vi "SPIM Controller.v2.vi"() -> ()   [LabVIEW 2015]
uses:
  controls/Microscope Settings.ctl
  controls/CameraState.ctl
  controls/Stack_State.ctl
  controls/Stack Track.ctl
  controls/CameraControlTypeDef.ctl
  controls/ModeEnum.ctl
  controls/Hardware.ctl
  <vilib>/Waveform/DWDTOps.llb/DWDT Append Digital Samples.vi
  <vilib>/Waveform/WDTOps.llb/WDT Append Waveforms DBL.vi
  <vilib>/Waveform/WDTOps.llb/WDT Waveform Duration DBL.vi
  <vilib>/vision/NI_Vision_Development_Module.lvlib
panel:
  out "Frames":i32
  out "Number Of Cameras":u32
  out "Numeric 3":i32
  out "Numeric 2":i32
  out "Stack Number":i32
  out "Numeric":i32
  in  "Tab Control":enum32{"Camera Settings", "Recording"}(tab)
  in  "Tweezers":T1={"Start /um"=40.0, "Step/um"=5.0, "Range /um"=20.0} {"Range /um" min=0.0 max=10.0 step=0.05; "Step/um" min=0.0001 max=10.0 step=0.05; "Start /um" min=0.0 max=10.0 step=0.05}
  in  "?":bool
  in  "Advanced DCAM Controls":i32(listbox) caption="Multicolumn Listbox"
  out "Waveform Duration":string
  in  "Microscope Settings":T2={"Mode"=enum."XY", "Slit"={"Scanning Mode"=12.0, "Slit Width /%"=5.0}, "Colour"=[{"Laser"=enum."561", "Filter"=4}], "Exposure/ms"=40.0, "Piezo Position /um"=0.0, "ROI"={"X"={"Start /px"=0.0, "Step /px"=1.0, "Range /px"=2048.0}, "Y"={"Start /px"=0.0, "Step /px"=1.0, "Range /px"=2048.0}, "Z "={"Start /um"=0.0, "Step/um"=1.0, "Range /um"=100.0}, "T "={"Start /s"=0.0, "Step /s"=1.0, "Range /s"=100.0}}, "Samples per millisecond"=100.0, "Relax/ms"=10.0, "Readout Direction"=2.0, "Trigger Source"=2.0, "Camera Delay /ms"=11.0, "Under Scan /ms"=5.0, "Calibration Coordinates"={"Top Left"=[-4.418670520231216, -0.1592138728323702, 10.0], "Top Right"=[-9.501965317919073, -0.1592138728323702, 10.0], "Bottom Left"=[-4.4508670520231215, 0.0, 0.0], "Bottom Right"=[-9.53757225433526, 0.0, 0.0], "Waveforms"={"Analogue Out"=[], "Digital Out"=[]}}} {"Under Scan /ms" min=0.0 max=10.0 step=0.05; "ROI"."T"."Range /s" min=0.0 max=10.0 step=0.05 format="%<%H:%M:%S>t"; "ROI"."T"."Step /s" min=0.0 max=10.0 step=0.05 format="%<%M:%S%2u>t"; "ROI"."T"."Start /s" min=0.0 max=10.0 step=0.05 format="%<%M:%S%2u>t"; "ROI"."X"."Range /px" min=0.0 max=10.0 step=0.05; "ROI"."X"."Step /px" min=0.0 max=10.0 step=0.05; "ROI"."X"."Start /px" min=0.0 max=10.0 step=0.05; "ROI"."Y"."Range /px" min=0.0 max=10.0 step=0.05; "ROI"."Y"."Step /px" min=0.0 max=10.0 step=0.05; "ROI"."Y"."Start /px" min=0.0 max=10.0 step=0.05; "ROI"."Z"."Range /um" min=0.0 max=10.0 step=0.05; "ROI"."Z"."Step/um" min=0.0001 max=10.0 step=0.05; "ROI"."Z"."Start /um" min=0.0 max=10.0 step=0.05; "Colour"."Filter" items=["Empty"=1, ""=2, ""=3, "561"=4, ""=5, "488"=6]; "Camera Delay /ms" min=0.0 max=10.0 step=0.05; "Trigger Source" items=["Internal"=1.0, "External"=2.0]; "Readout Direction" items=["Forward"=1.0, "Backward"=2.0]; "Slit"."Scanning Mode" items=["Full Frame"=1.0, "Slit Scanning"=12.0]; "Piezo Position /um" min=0.0 max=10.0 step=0.05}
  in  "Frames":i32
  in  "Scan Continuously":bool
  in  "Scan Cont":bool
  in  "Scans":dbl=1.0 min=0.0 max=10.0 step=0.05
  in  "Scan":bool
  in  "Save to:":path=path "C:/_DATA/test.tiff"
  out "error IO":errorcluster
  in  "Multicolumn Listbox":i32(listbox)
  out "FPS":dbl
  out "Image":T3(plugin-control)
  out "Histogram":T4(graph)
  in  "stop":bool
  in  "Load Settings":bool
  in  "Save Settings":bool
  in  "Record":bool
  in  "Signals Debugger":bool
  in  "Stage Controller":bool
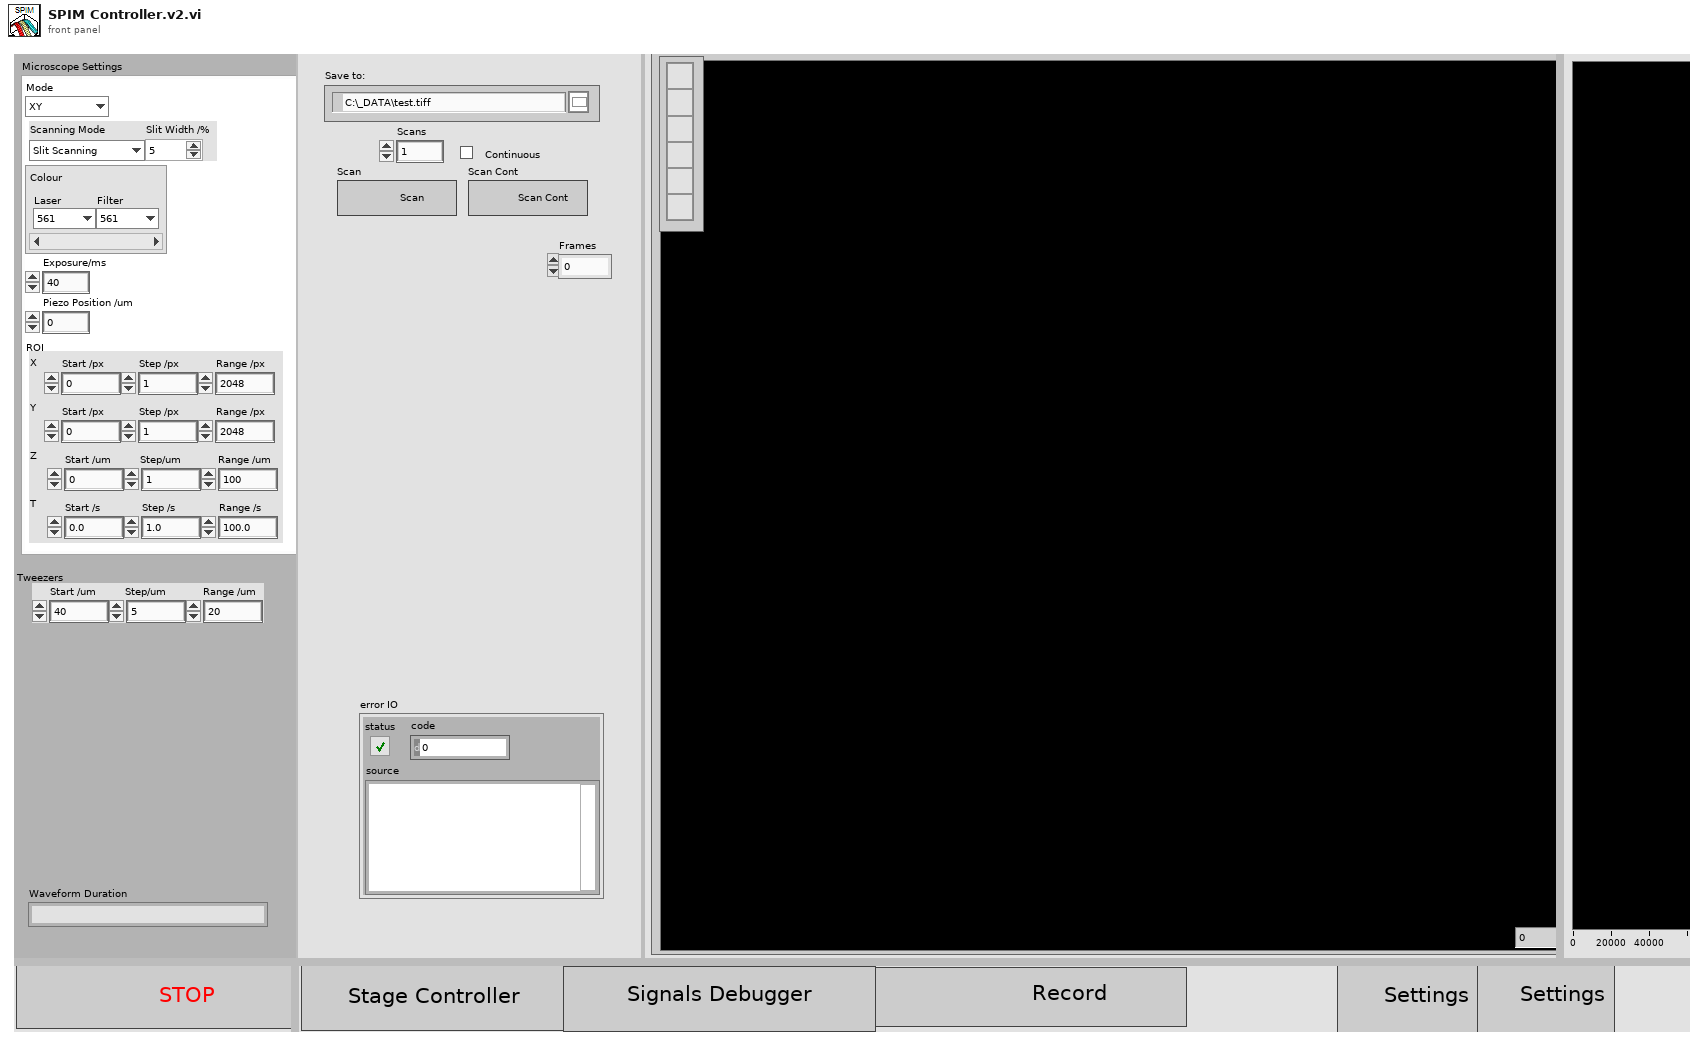
[diagram p1: front panel]
types:
  T1 = cluster{"Start /um":dbl, "Step/um":dbl, "Range /um":dbl}
  T2 = typedef "Microscope Settings.ctl" = cluster{"Mode":enum16{"X", "XY", "XYZ", "XYZT", "XYZC", "Tweezers", "Virus"}, "Slit":cluster{"Scanning Mode":dbl, "Slit Width /%":dbl}, "Colour":cluster{"Laser":enum16{"Brightfield", "445", "488", "561", "647"}, "Filter":u16}[], "Exposure/ms":dbl, "Piezo Position /um":dbl, "ROI":cluster{"X":cluster{"Start /px":dbl, "Step /px":dbl, "Range /px":dbl}, "Y":cluster{"Start /px":dbl, "Step /px":dbl, "Range /px":dbl}, "Z ":cluster{"Start /um":dbl, "Step/um":dbl, "Range /um":dbl}, "T ":cluster{"Start /s":dbl, "Step /s":dbl, "Range /s":dbl}}, "Samples per millisecond":dbl, "Relax/ms":dbl, "Readout Direction":dbl, "Trigger Source":dbl, "Camera Delay /ms":dbl, "Under Scan /ms":dbl, "Calibration Coordinates":cluster{"Top Left":dbl[], "Top Right":dbl[], "Bottom Left":dbl[], "Bottom Right":dbl[], "Waveforms":cluster{"Analogue Out":waveform(dbl)[], "Digital Out":digitalwaveform[]}}}
  T3 = typedef "IMAQ Image.ctl" = refnum<image>
  T4 = cluster{"Starting Value":sgl, "Incremental Value":sgl, "Histogram":u32[]}
  T5 = cluster{"height":u32, "width":u32, "datatype":u32}
  T6 = typedef "CameraState.ctl" = enum16{"init", "active", "deinit"}
  T7 = cluster{"Mode":u32, "Polarity":u32, "Times":u32, "Delay":dbl}
  T8 = typedef "Stack_State.ctl" = cluster{"State":T9, "Stack Number":i32, "Image":u16[][], "Stacks":i32}
  T9 = typedef "Stack Track.ctl" = enum16{"Idle", "Display", "Start Sequence", "Read Disk", "STOP", "Collecting", "End", "Save Image"}
  T10 = typedef "ModeEnum.ctl" = enum16{"Idle", "generateWaves", "runWaves", "runWavesCont", "endWavesCont", "stop"}
  T11 = typedef "CameraControlTypeDef.ctl" = enum16{"Idle", "IntervalLineInt", "Ram Record", "HardDisk Record", "Disengage Update", "Update", "ROI", "Binning", "Scan Mode", "Trigger Mode", "Readout Mode", "Readout Direction", "Preview", "ROIWindow", "Trigger Source"}
  T12 = typedef "Hardware.ctl" = enum16{"Stop", "RunCont", "EndCont", "Idle", "Update", "Run Waves"}
  T13 = cluster{"Laser":enum16{"Brightfield", "445", "488", "561", "647"}, "Filter":u16}[]
  T14 = enum32{"Invalid", "Standard", "Closed", "Hidden", "Minimized", "Maximized"}
  T15 = enum16{"open", "replace", "create", "open or create", "replace or create", "replace or create with confirmation"}
  T16 = typedef "Image Type" = u32
  T17 = enum16{"X", "XY", "XYZ", "XYZT", "XYZC", "Tweezers", "Virus"}
  T18 = cluster{"Analogue Out out":waveform(dbl)[], "Digital Out out":digitalwaveform[]}
  T19 = cluster{"State":T9, "Timeout":i32, "Data 16":u16[][], "Timeout":i32}
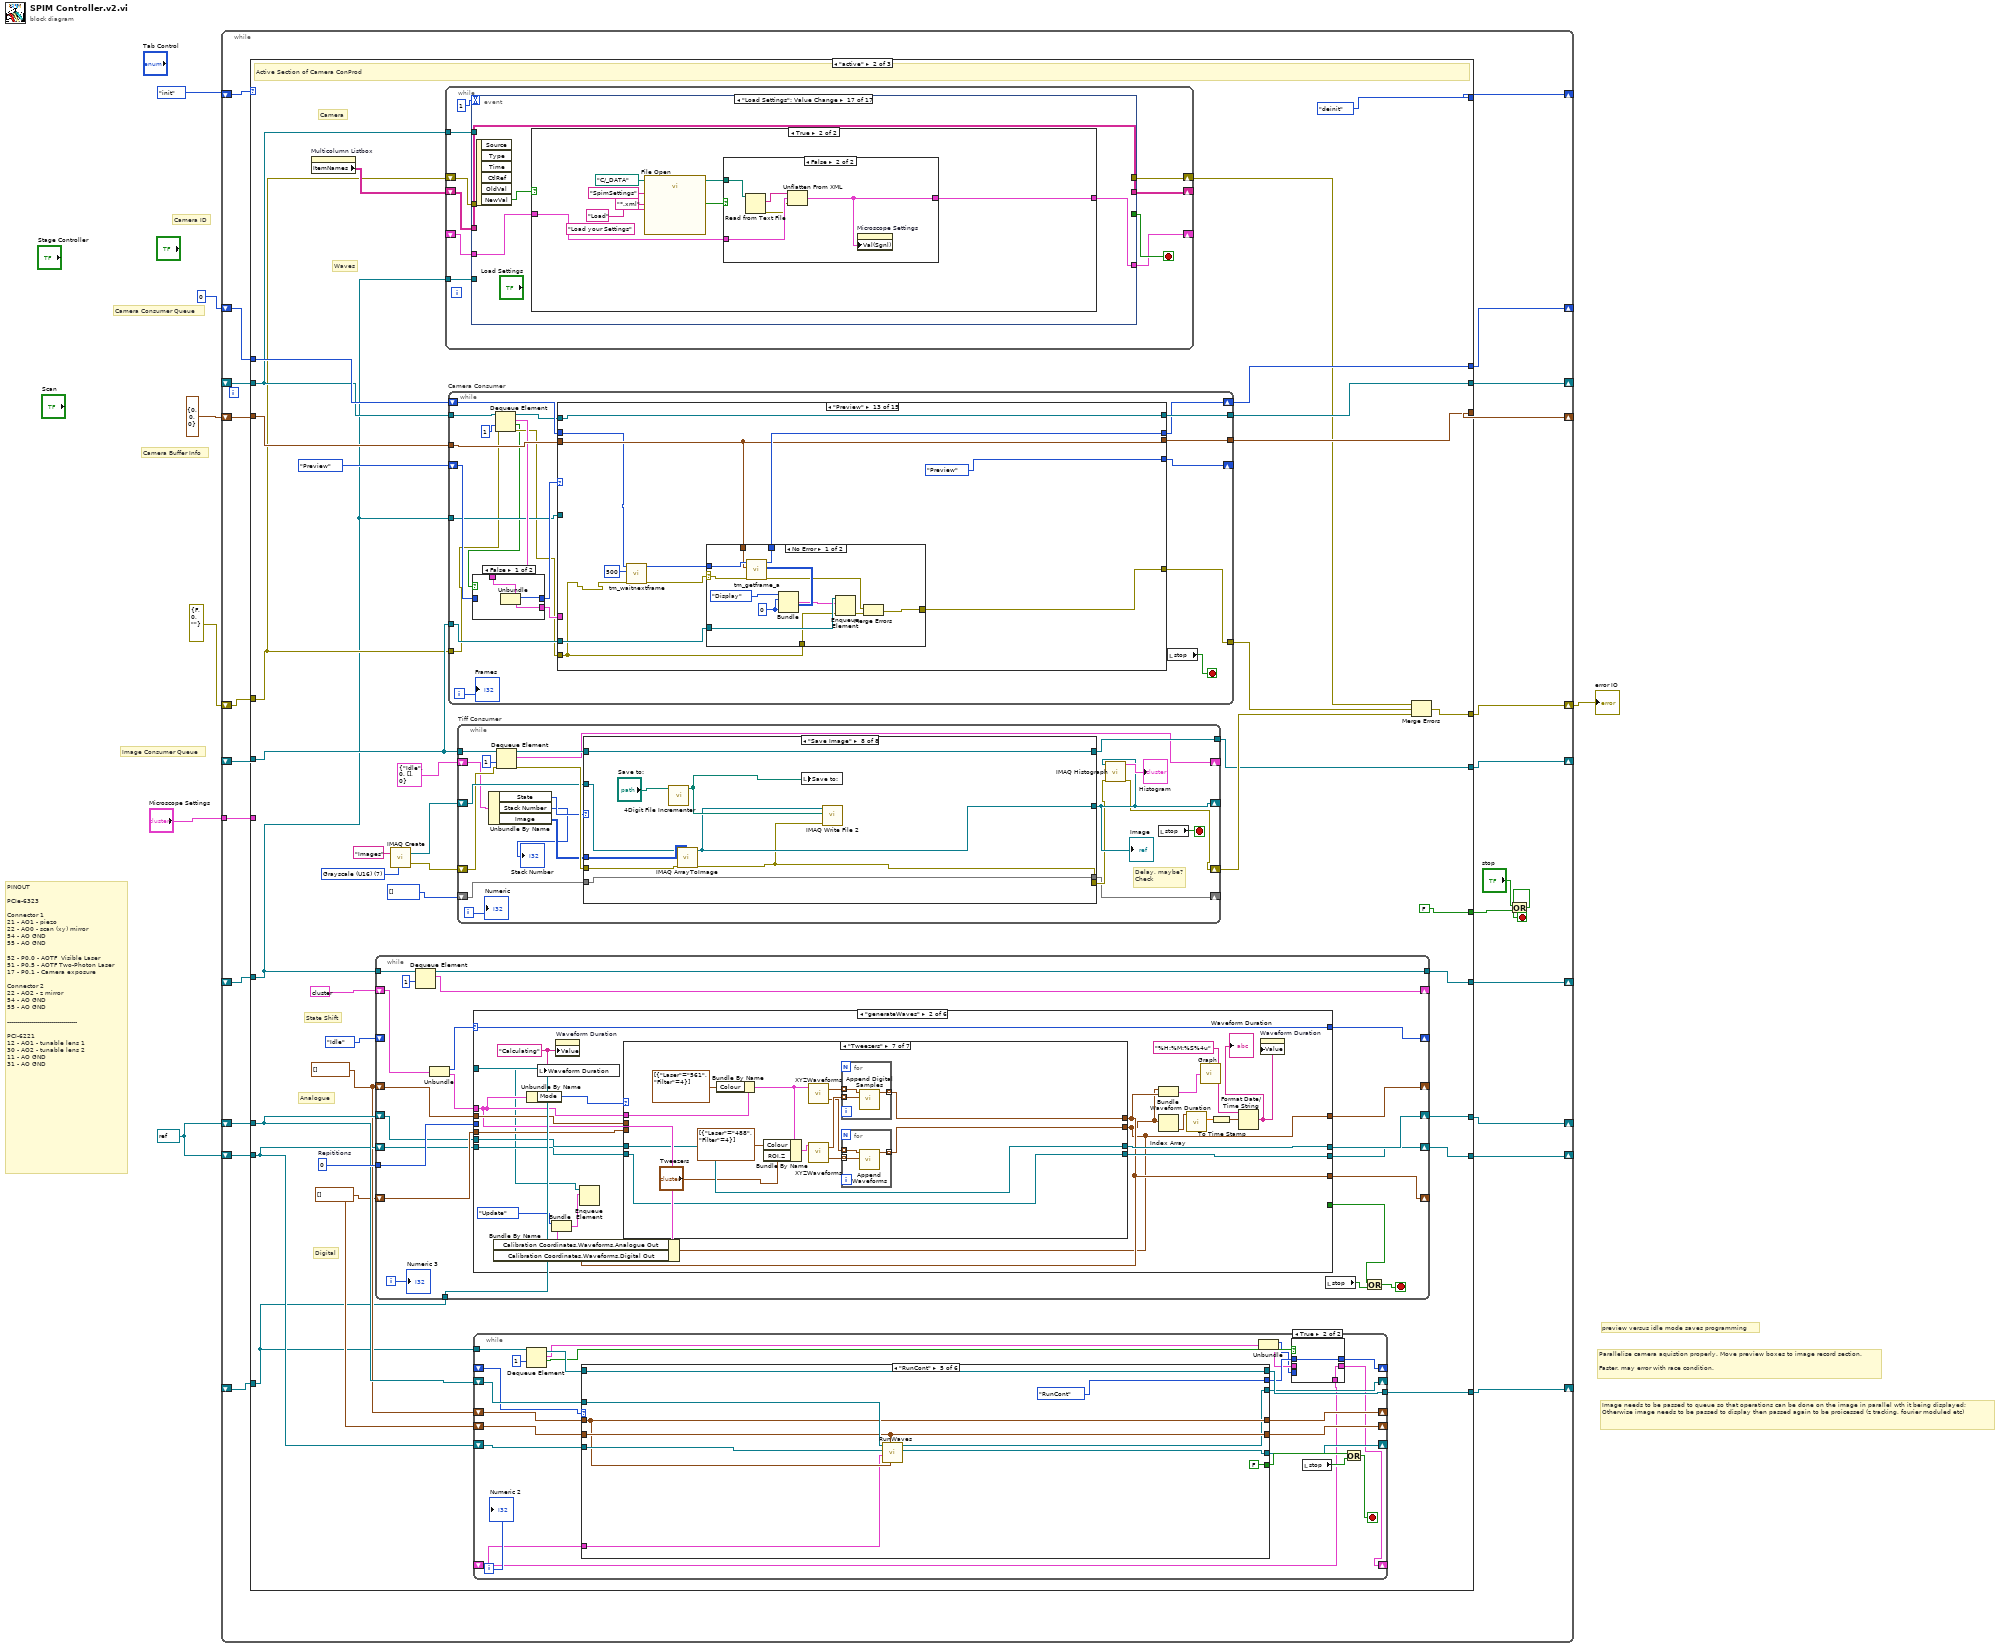
[diagram p0: block diagram]
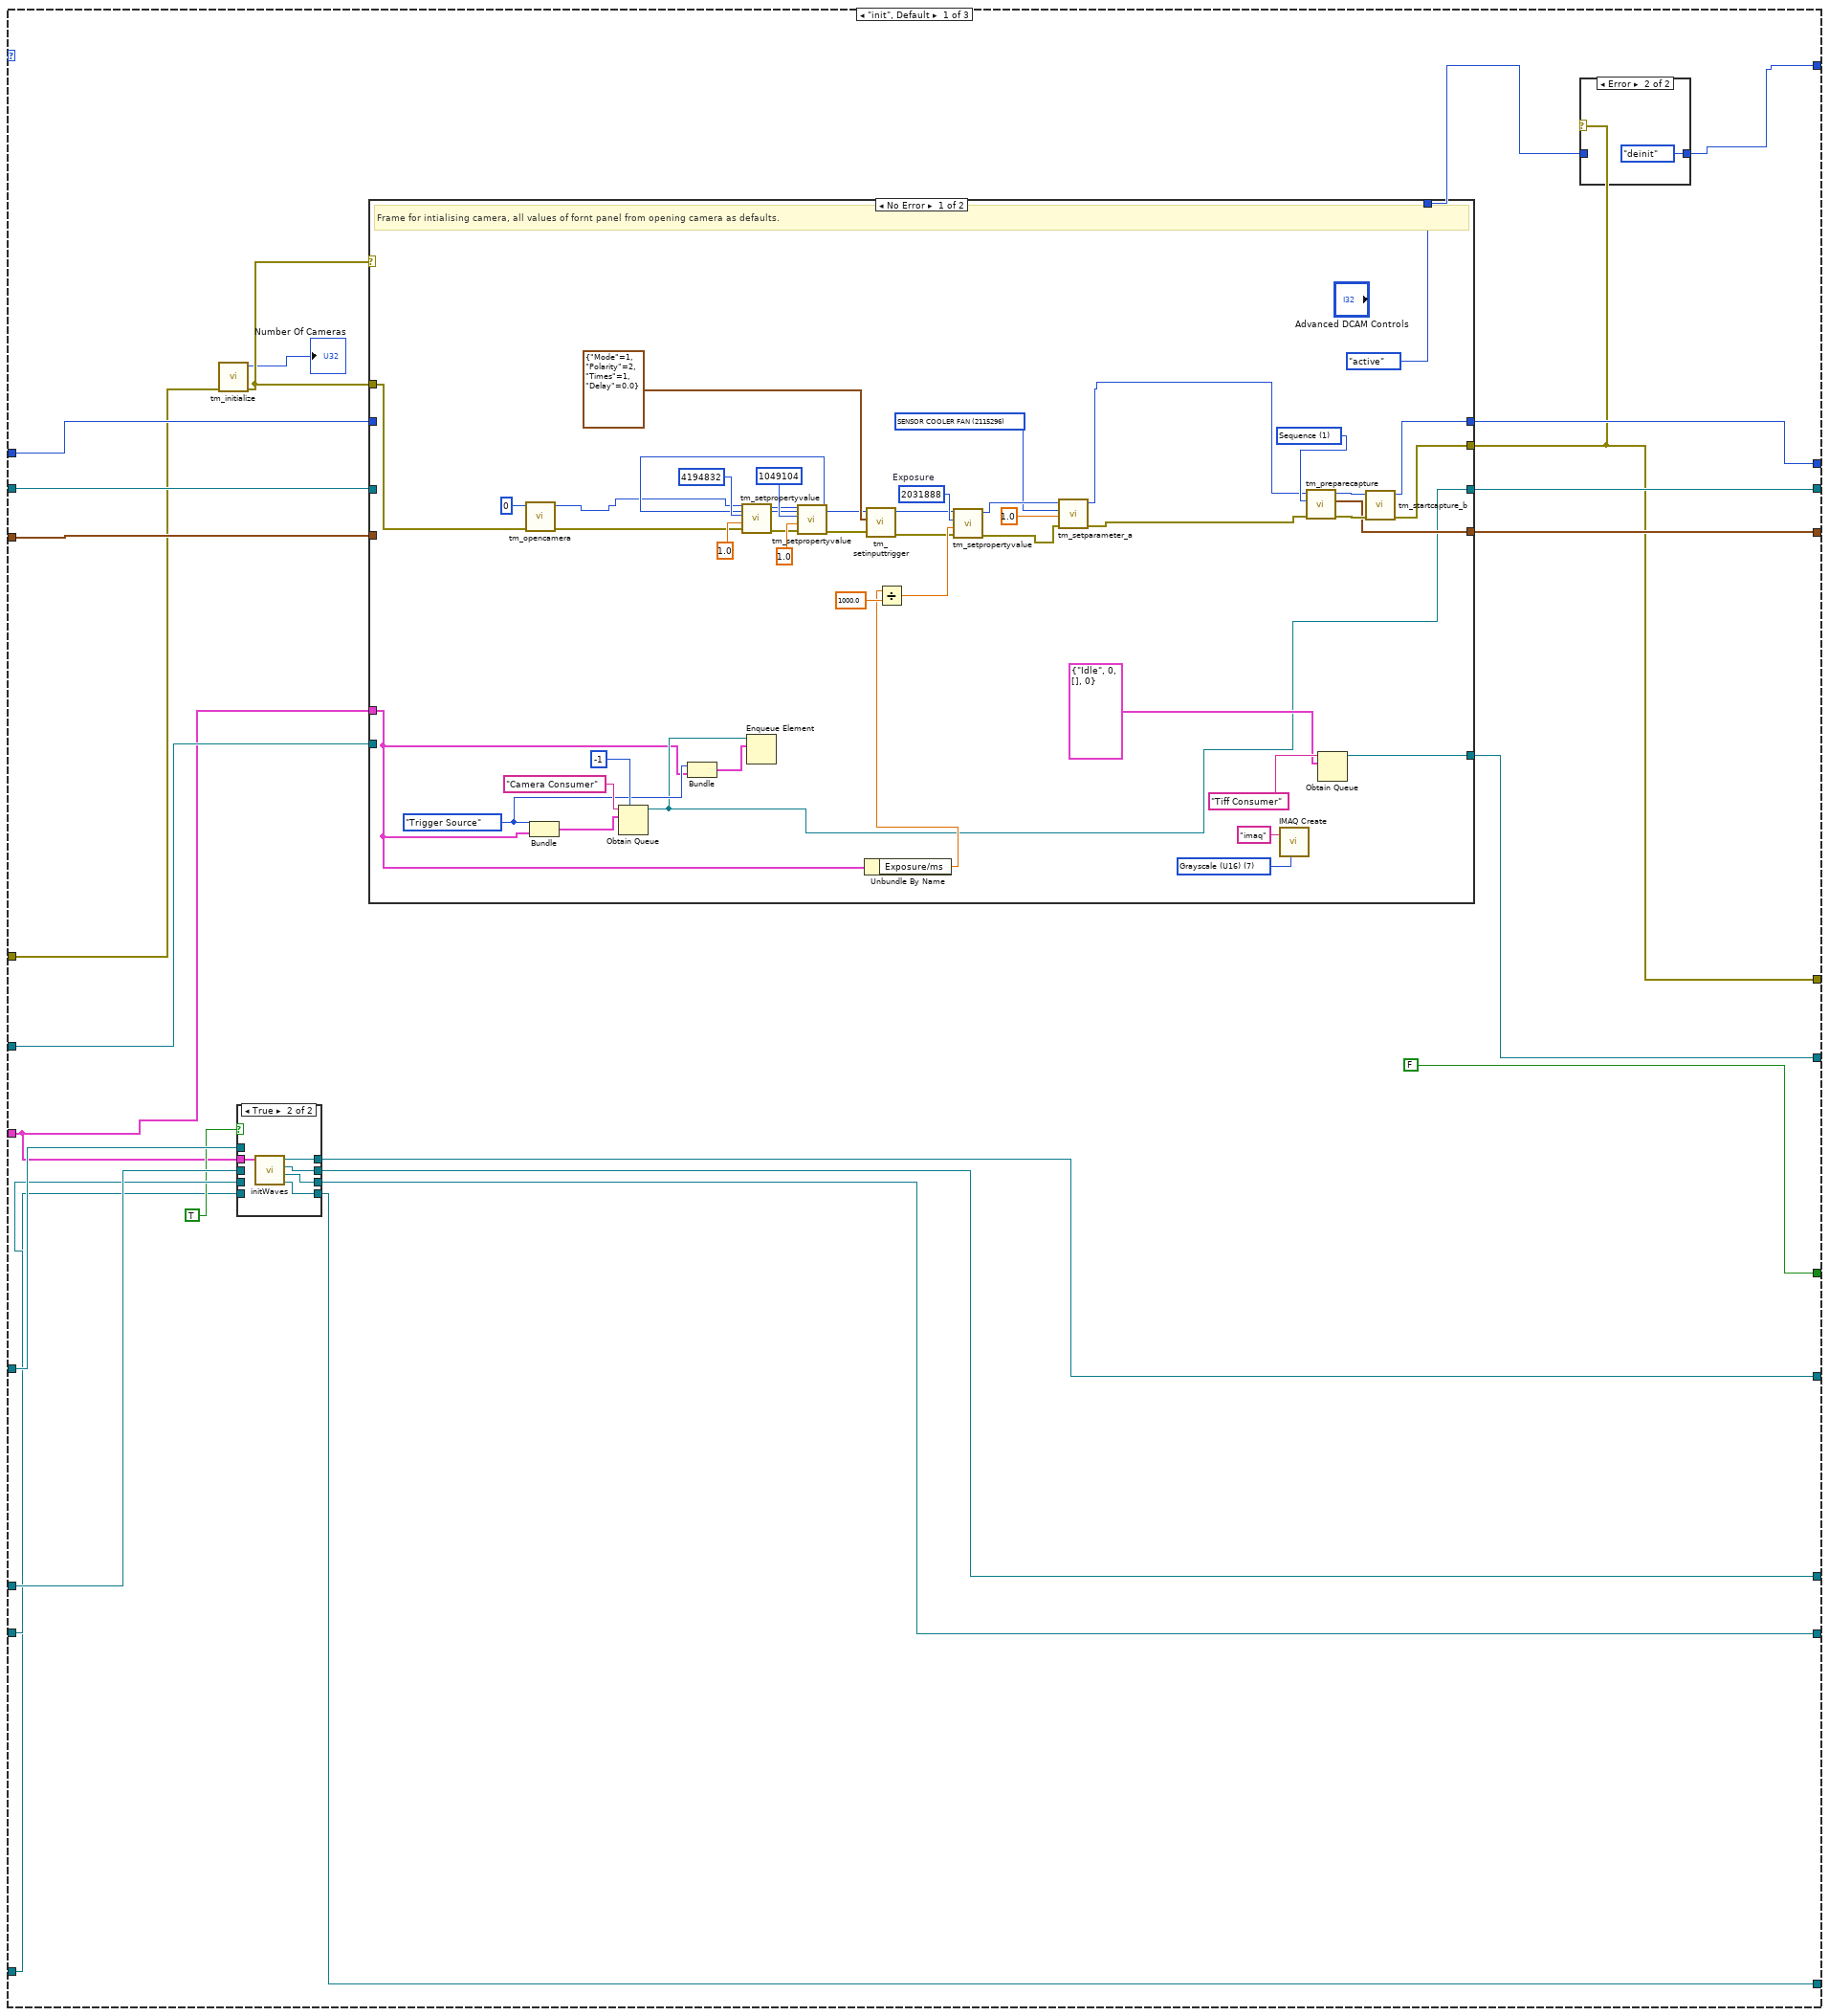
[diagram p2: hidden frame]
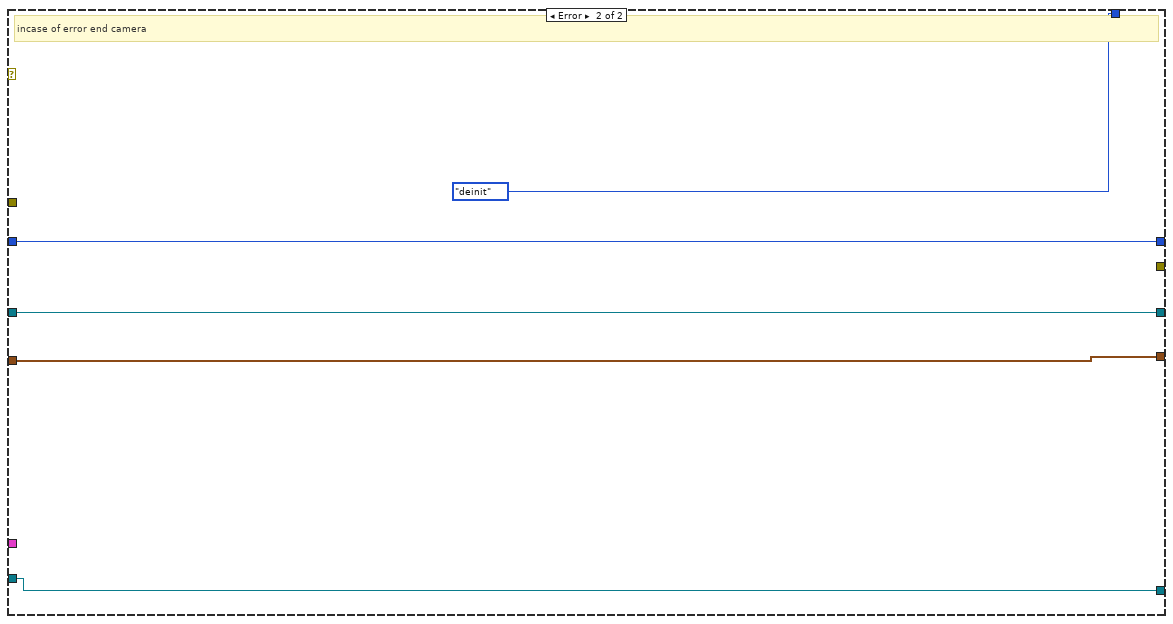
[diagram p5: hidden frame]
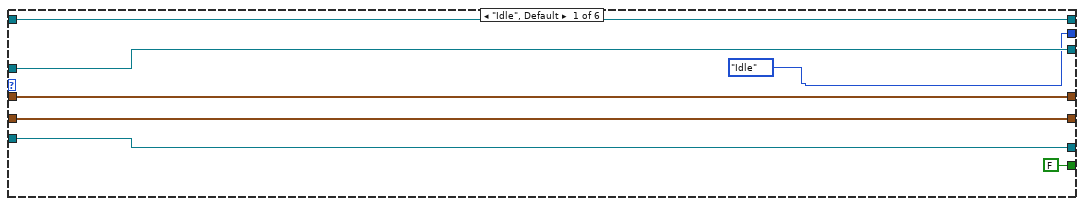
[diagram p7: hidden frame]
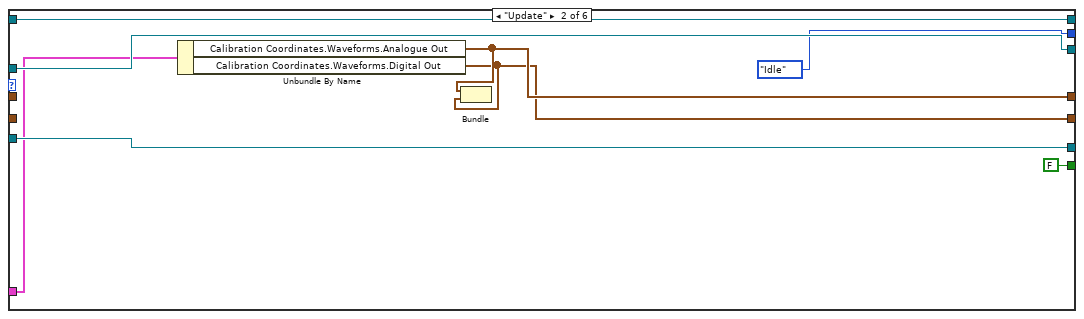
[diagram p8: hidden frame]
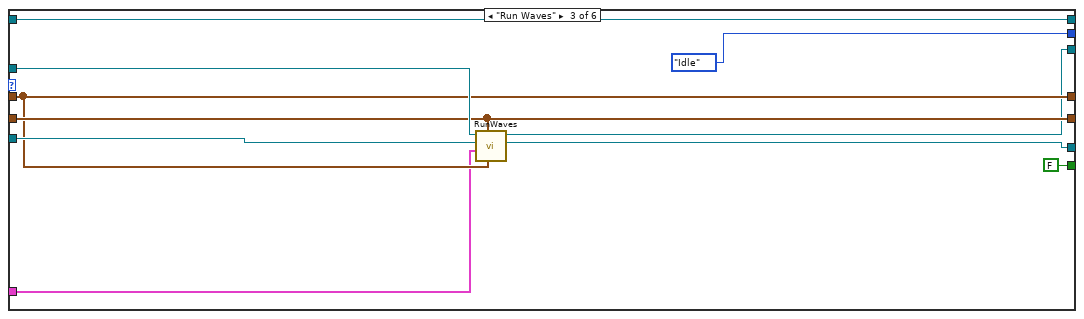
[diagram p9: hidden frame]
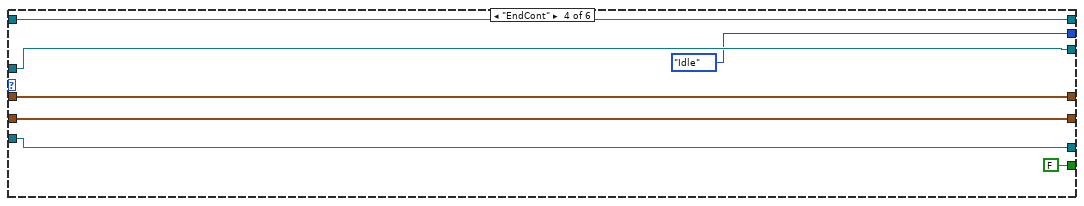
[diagram p10: hidden frame]
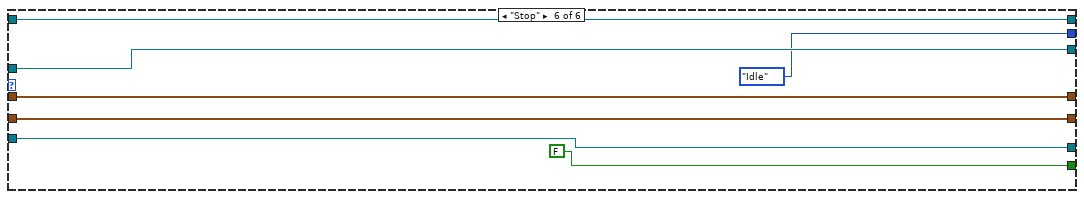
[diagram p11: hidden frame]
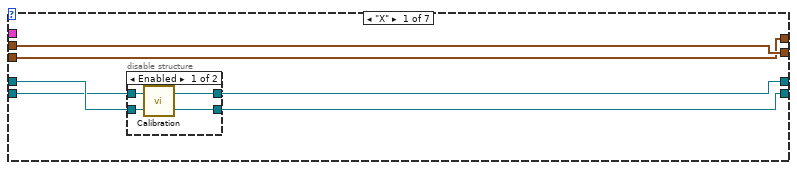
[diagram p13: hidden frame]
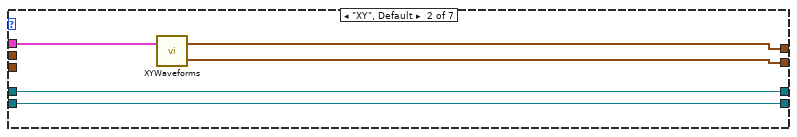
[diagram p15: hidden frame]
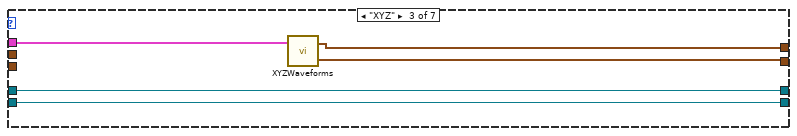
[diagram p16: hidden frame]
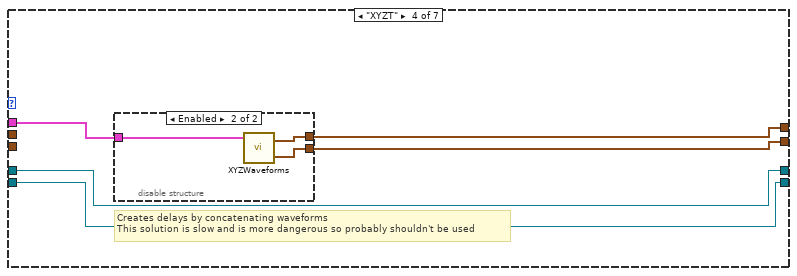
[diagram p17: hidden frame]
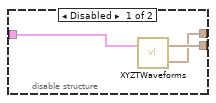
[diagram p18: hidden frame]
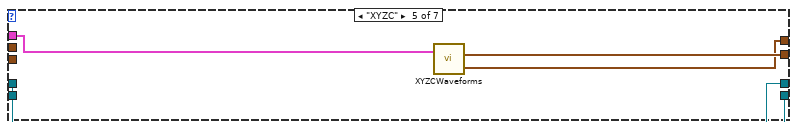
[diagram p19: hidden frame]
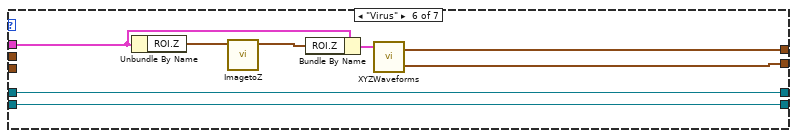
[diagram p20: hidden frame]
diagram:
  w4 = refnum<k21> refnum ("Mirror Z 2")
  # "PINOUT\n\nPCIe-6323\n\nConnector 1\n21 - AO1 - piezo\n22 - AO0 - scan (xy) mirror\n54 - AO GND\n55 - AO GND\n\n52 - P0.0 - AOTF  Visible Laser\n51 - P0.5 - AOTF Two-Photon Laser\n17 - P0.1 - Camera exposure\n\nConnector 2\n22 - AO2 - z mirror\n54 - AO GND\n55 - AO GND\n\n-----------------------------------\n\nPCI-6221\n12 - AO1 - tunable lens 1\n30 - AO2 - tunable lens 2\n11 - AO GND\n31 - AO GND"
  # "Camera Buffer Info"
  # "Image needs to be passed to queue so that operations can be done on the image in parallel wth it being displayed;\nOtherwise image needs to be passed to display then passed again to be proicessed (z tracking, fourier moduled etc)"
  # "preview versus idle mode saves programming"
  # "Parallelise camera aquistion properly. Move preview boxes to image record section.\n\nFaster. may error with race condition."
  # "Image Consumer Queue"
  # "Camera Consumer Queue"
  # "Camera ID"
  n1 = while {
    shift-right: [w31] -> _
    shift-left: CameraState."init" -> [w9]
    shift-right: [w30] -> _
    shift-left: u32 0 ("Handle out") -> [w29]
    shift-right: [w28] -> w6
    shift-left: errorcluster {"status"=FALSE, "code"=0, "source"=""} ("error IO") -> [w27]
    shift-right: [w26] -> _
    shift-left: _ -> [w25]
    shift-right: [w12] -> _
    shift-left: _ -> [w24]
    shift-right: [w20] -> _
    shift-left: T5 {"height"=0, "width"=0, "datatype"=0} ("Buffer Info") -> [w19]
    shift-right: [w18] -> _
    shift-left: w4 -> [w17]
    shift-right: [w15] -> _
    shift-left: w4 -> [w16]
    shift-right: [w14] -> _
    shift-left: _ -> [w13]
    shift-right: [w11] -> _
    shift-left: _ -> [w10]
    tunnel: "Microscope Settings" -> [w8]
    stop <- w22 stop-if-true
    n2 = case shown="\"active\"" w9 {
      tunnel: [w33 CameraState."deinit" CameraState."init"] -> w31
      tunnel: [w56 w151 w911] -> w30
      tunnel: w29 -> [w47 w152 w911]
      tunnel: [w35 w150 w914] -> w28
      tunnel: w27 -> [w45 w132 w915]
      tunnel: [w55 w147 w899] -> w12
      tunnel: [w54 w146 w895] -> w26
      tunnel: w25 -> [w52 w140 w895]
      tunnel: w24 -> [w53 w139 w899]
      tunnel: [FALSE ("stop") FALSE ("stop") TRUE ("stop")] -> w21
      tunnel: [w50 w143 w908] -> w20
      tunnel: w19 -> [w49 w142 w908]
      tunnel: w13 -> [w42 w126 w894]
      tunnel: [w48 w136 w906] -> w18
      tunnel: w17 -> [w41 w125 w906]
      tunnel: w16 -> [w40 w124 w904]
      tunnel: [w46 w137 w904] -> w15
      tunnel: [w43 w135 w894] -> w14
      tunnel: [w38 w121 w893] -> w11
      tunnel: w10 -> [w37 w120 w893]
      tunnel: w8 -> [w36 _ _]
      frame "init", Default {
        n3 = call "tm_initialize.vi"("error in (no error)"=w45) -> ("error out"=w44:errorcluster, "Number Of Cameras"=→"Number Of Cameras":u32)  [unwired: 7 in, 2 out]
        n4 = case shown="True" TRUE {
          tunnel: [w61 w67] -> w48
          tunnel: [w60 w65] -> w46
          tunnel: w36 -> [_ w63]
          tunnel: [w62 w66] -> w43
          tunnel: w42 -> [w62 _]
          tunnel: w41 -> [w61 _]
          tunnel: w40 -> [w60 _]
          tunnel: [w59 w64] -> w38
          tunnel: w37 -> [w59 _]
          frame False {
          }
          frame True {
            n5 = call "initWaves.vi"("Microscope Settings"=w63) -> ("Waveform Player"=w64:refnum<queue>, "Digital"=w65:refnum<k21>, "Analogue"=w67:refnum<k21>, "Waveform Controller"=w66:refnum<queue>)  [unwired: 4 in]
          }
        }
        n6 = case shown="No Error" w44 {
          tunnel: w44 -> [w86 _]
          tunnel: [CameraState."active" CameraState."deinit"] -> w34
          tunnel: [w108 _] -> w35
          tunnel: [w106 w112] -> w56
          tunnel: [w74 w115] -> w55
          tunnel: [w103 w114] -> w54
          tunnel: w53 -> [_ w115]
          tunnel: w52 -> [_ w114]
          tunnel: [w101 w113] -> w50
          tunnel: w49 -> [_ w113]
          tunnel: w47 -> [_ w112]
          tunnel: w36 -> [w73 _]
          frame No Error {
            w83 = u32 2115296 items=["SENSOR MODE"=4212128, "CCD MODE"=4212384, "READOUT MODE"=4211872, "ACTIVE VIEW INDEX"=4343136, "BITS PER CHANNEL"=4342976, "IMAGE PIXEL TYPE"=4343296, "BINNING"=4215968, "EXPOSURE TIME"=2049184, "CONTRAST GAIN"=3163312, "CONTRAST OFFSET"=3163328, "LIGHT MODE"=2114720, "SENSITIVITY"=2114992, "PHOTON IMAGING MODE"=2115200, "HIGH DYNAMIC RANGE MODE"=3163360, "WHITE BALANCE"=3163568, "TEMPERATURE"=2115232, "TEMPERATURE TARGET"=2115264, "SENSOR COOLER FAN"=2115296, "LINEBUNDLE HEIGHT"=4212192, "MECHANICAL SHUTTER"=2115488, "BACK FOCUS POSITION"=8422304, "TRIGGER CONNECTOR"=1066432, "TRIGGER SOURCE"=1066144, "OUTPUT TRIGGER SOURCE"=1852576, "TRIGGER GLOBAL EXPOSURE"=2049680, "FIRST TRIGGER BEHAVIOR"=2049696, "CHANNEL SYNC"=1852352, "READOUT DIRECTION"=4211904, "PRE HSYNC COUNT"=1852704, "INTERNAL LINE SPEED"=4226000, "INTERNAL LINE INTERVAL"=4226016] ("Parameter")
            w76 = CameraControlTypeDef."Trigger Source" ("Enum")
            w90 = u32 2031888  # Exposure
            w100 = T16 7 items=["Grayscale (U8)", "Grayscale (I16)", "Grayscale (SGL)", "Complex (CSG)", "RGB (U32)", "HSL (U32)", "RGB (U64)", "Grayscale (U16)"] ("Image Type")
            w110 = 1 items=["Snap", "Sequence"] ("Capture mode")
            # "Frame for intialising camera, all values of fornt panel from opening camera as defaults."
            n7 = call "tm_opencamera.vi"("error in (no error)"=w86, "Camera Index"=u32 0) -> ("error out"=w68:errorcluster, "Handle out"=w69:u32)  [unwired: 7 in, 1 out]
            n8 = Bundle("Enum"=w76, "Microscope Settings"=w73) -> (w75:cluster{"Enum":T11, "Microscope Settings":T2})  [unwired: 1 in]
            n9 = Obtain Queue(max queue size (-1, unlimited)=-1, name (unnamed)="Camera Consumer", element data type=w75) -> (queue out=w74:refnum<queue>)  [unwired: 2 in, 2 out]
            n10 = Bundle("Enum"=w76, "Microscope Settings"=w73) -> (w72:cluster{"Enum":T11, "Microscope Settings":T2})  [unwired: 1 in]
            n11 = call "tm_setpropertyvalue.vi"("error in (no error)"=w68, "Value in"=sgl 1.0, "Property ID"=u32 4194832, "Handle in"=w69) -> ("error out"=w80:errorcluster, "Handle out"=w93:u32)  [unwired: 6 in]
            n12 = Enqueue Element(queue=w74, element=w72) -> ()  [unwired: 2 in, 3 out]
            n13 = call "tm_setpropertyvalue.vi"("error in (no error)"=w80, "Value in"=sgl 1.0, "Property ID"=u32 1049104, "Handle in"=w93) -> ("error out"=w79:errorcluster, "Handle out"=w91:u32)  [unwired: 6 in]
            n14 = Unbundle By Name(w73) -> ("Exposure/ms"=w81:dbl)
            n15 = call "tm_setinputtrigger.vi"("error in (no error)"=w79, "Parameters"=T7 {"Mode"=1, "Polarity"=2, "Times"=1, "Delay"=0.0}, "Handle in"=w91) -> ("error out"=w78:errorcluster, "Handle out"=w89:u32)  [unwired: 7 in]
            n16 = Divide(x=w81, y=sgl 1000.0) -> (x/y=w87:dbl)
            n17 = call "tm_setpropertyvalue.vi"("error in (no error)"=w78, "Value in"=w87, "Property ID"=w90, "Handle in"=w89) -> ("error out"=w77:errorcluster, "Handle out"=w84:u32)  [unwired: 6 in]
            n18 = call "tm_setparameter_a.vi"("error in (no error)"=w77, "Value in"=1.0, "Parameter"=w83, "Handle in"=w84) -> ("error out"=w70:errorcluster, "Handle out"=w71:u32)  [unwired: 6 in]
            n19 = call "IMAQ Create"("Image Name"="imaq", "Image Type"=w100) -> ()  [unwired: 3 in, 2 out]
            n20 = call "tm_preparecapture.vi"("error in (no error)"=w70, "Capture mode"=w110, "Handle in"=w71) -> ("error out"=w109:errorcluster, "Buffer Info"=w101:T5, "Handle out"=w107:u32)  [unwired: 5 in, 1 out]
            n21 = Obtain Queue(name (unnamed)="Tiff Consumer", element data type=T8 {"State"=enum."Idle", "Stack Number"=0, "Image"=[], "Stacks"=0} ("input cluster")) -> (queue out=w103:refnum<queue>)  [unwired: 3 in, 2 out]
            n22 = call "tm_startcapture_b.vi"("error in (no error)"=w109, "Handle in"=w107) -> ("error out"=w108:errorcluster, "Handle out"=w106:u32)  [unwired: 8 in]
          }
          frame Error {
            # "incase of error end camera"
          }
        }
        n23 = case shown="Error" w35 {
          tunnel: [w57 CameraState."deinit"] -> w33
          tunnel: w34 -> [w57 _]
          frame No Error {
          }
          frame Error {
          }
        }
      }
      frame "active" {
        w119 = T16 7 items=["Grayscale (U8)", "Grayscale (I16)", "Grayscale (SGL)", "Complex (CSG)", "RGB (U32)", "HSL (U32)", "RGB (U64)", "Grayscale (U16)"] ("Image Type")
        w122 = digitalwaveform[] [] ("Digital Out")
        w123 = waveform(dbl)[] [] ("Analogue Out")
        w138 = 0  # Repititions
        # "State Shift"
        # "Waves"
        # "Camera"
        # "Digital"
        # "Analogue"
        # "Active Section of Camera ConProd"
        n24 = property on="Multicolumn Listbox" class="MCListbox (strict)"() -> ("ItemNames"=w134:string[][])  [unwired: 2 in, 2 out]
        n25 = while {
          tunnel: w126 -> [w252]
          shift-right: [w251] -> _
          shift-left: w123 -> [w250]
          tunnel: w138 -> [w249]
          shift-right: [w245] -> w136
          shift-left: w125 -> [w244]
          shift-right: [w248] -> _
          shift-left: w122 -> [w247]
          shift-right: [w243] -> w137
          shift-left: w124 -> [w242]
          tunnel: [w241] -> w135
          shift-right: [w237] -> _
          shift-left: ModeEnum."Idle" ("Mode") -> [_]
          tunnel: w120 -> [w234]
          shift-right: [w232] -> _
          shift-left: cluster{"Mode":T10, "Microscope Settings":T2} {"Mode"=enum."Idle", "Microscope Settings"={"Mode"=enum."X", "Slit"={"Scanning Mode"=0.0, "Slit Width /%"=0.0}, "Colour"=[], "Exposure/ms"=0.0, "Piezo Position /um"=0.0, "ROI"={"X"={"Start /px"=0.0, "Step /px"=0.0, "Range /px"=0.0}, "Y"={"Start /px"=0.0, "Step /px"=0.0, "Range /px"=0.0}, "Z "={"Start /um"=0.0, "Step/um"=0.0, "Range /um"=0.0}, "T "={"Start /s"=0.0, "Step /s"=0.0, "Range /s"=0.0}}, "Samples per millisecond"=0.0, "Relax/ms"=0.0, "Readout Direction"=0.0, "Trigger Source"=0.0, "Camera Delay /ms"=0.0, "Under Scan /ms"=0.0, "Calibration Coordinates"={"Top Left"=[], "Top Right"=[], "Bottom Left"=[], "Bottom Right"=[], "Waveforms"={"Analogue Out"=[], "Digital Out"=[]}}}} -> [w231]
          i -> [w233]
          stop <- w238 stop-if-true
          n26 = Dequeue Element(queue=w252, timeout in ms (-1)=1) -> (queue out=w241:refnum<queue>, element=w232:cluster{"Mode":T10, "Microscope Settings":T2})  [unwired: 1 in, 2 out]
          n27 = Unbundle(w231) -> ("Mode"=w236:T10, "Microscope Settings"=w235:T2)
          n28 = case shown="\"generateWaves\"" w236 {
            selector: w236 -> [w253 w266 w352 w361 w371 w374]
            tunnel: [_ _ _ _ FALSE TRUE] -> w240
            tunnel: w235 -> [_ w265 w348 w357 w367 _]
            tunnel: [w257 w261 w350 w359 w369 w379] -> w251
            tunnel: w250 -> [w257 w277 w350 w359 w369 w379]
            tunnel: w249 -> [_ _ _ _ _ _]
            tunnel: [w254 w267 w354 w363 w373 w378] -> w243
            tunnel: [w255 w269 w353 w362 w372 w377] -> w245
            tunnel: w244 -> [w255 w270 w353 w362 w372 w377]
            tunnel: [w256 w262 w349 w358 w368 w376] -> w248
            tunnel: w247 -> [w256 w279 w349 w358 w368 w376]
            tunnel: w242 -> [w254 w268 w354 w363 w373 w378]
            tunnel: [w253 w266 w352 w361 w371 w374] -> w237
            tunnel: w234 -> [_ w263 w351 w360 w370 _]
            frame "Idle", Default {
            }
            frame "generateWaves" {
              w272 = "Calculating" ("date/time string")
              n29 = Unbundle By Name(w265) -> ("Mode"=w278:T17)
              n30 = local write "Waveform Duration"(w272) -> ()
              n31 = property on="Waveform Duration" class="Str"("Value"=w272) -> ()  [unwired: 2 in, 2 out]
              n32 = case shown="\"Tweezers\"" w278 {
                tunnel: [w285 w295 w298 w306 w317 w322 w327] -> w261
                tunnel: w265 -> [_ w296 w299 w304 w313 w321 w336]
                tunnel: [w284 w294 w297 w305 w316 w323 w330] -> w262
                tunnel: w279 -> [w284 _ _ _ _ _ _]
                tunnel: w277 -> [w285 _ _ _ _ _ _]
                tunnel: w270 -> [w283 w293 w301 w303 w315 w325 w339]
                tunnel: w268 -> [w282 w292 w300 w302 w314 w324 w338]
                tunnel: [w281 w293 w301 w303 w315 w325 w339] -> w269
                tunnel: [w280 w292 w300 w302 w314 w324 w338] -> w267
                frame "X" {
                  n33 = disable-structure shown="Enabled" {
                    disable-tunnel: w283 -> [w289 w290]
                    disable-tunnel: w282 -> [w288 w291]
                    disable-tunnel: [w287 w291] -> w281
                    disable-tunnel: [w286 w290] -> w280
                    frame Enabled {
                      n34 = call "Calibration.vi"("Analogue In"=w289, "Digital In"=w288) -> ("Analogue In Out"=w286:refnum<k21>, "Digital Out"=w287:refnum<k21>)
                    }
                    frame Disabled {
                    }
                  }
                }
                frame "XY", Default {
                  n35 = call "XYWaveforms.vi"("Microscope Settings"=w296) -> ("Analogue Out"=w295:waveform(dbl)[], "Digital Out"=w294:digitalwaveform[])  [unwired: 1 out]
                }
                frame "XYZ" {
                  n36 = call "XYZWaveforms.vi"("Microscope Settings"=w299) -> ("Analogue Out out"=w298:waveform(dbl)[], "Digital Out out"=w297:digitalwaveform[])  [unwired: 2 in]
                }
                frame "XYZT" {
                  # "Creates delays by concatenating waveforms\nThis solution is slow and is more dangerous so probably shouldn't be used"
                  n37 = disable-structure shown="Enabled" {
                    disable-tunnel: [w309 w310] -> w306
                    disable-tunnel: [w308 w311] -> w305
                    disable-tunnel: w304 -> [w307 w312]
                    frame Disabled {
                      n38 = call "XYZTWaveforms.vi"("Microscope Settings"=w307) -> ("Digital Out"=w308:digitalwaveform[], "Analogue Out"=w309:waveform(dbl)[])  [unwired: 1 in]
                    }
                    frame Enabled {
                      n39 = call "XYZWaveforms.vi"("Microscope Settings"=w312) -> ("Analogue Out out"=w310:waveform(dbl)[], "Digital Out out"=w311:digitalwaveform[])  [unwired: 2 in]
                    }
                  }
                }
                frame "XYZC" {
                  n40 = call "XYZCWaveforms.vi"("Microscope Settings"=w313) -> ("Array"=w316:digitalwaveform[], "Analogue Out out"=w317:waveform(dbl)[])  [unwired: 1 in]
                }
                frame "Virus" {
                  n41 = Unbundle By Name(w321) -> ("ROI.Z"=w319:T1)
                  n42 = call "ImagetoZ.vi"("Z"=w319) -> ("ROI.Z"=w318:T1)  [unwired: 10 in]
                  n43 = Bundle By Name(cluster=w321, "ROI.Z"=w318) -> (w320:T2)
                  n44 = call "XYZWaveforms.vi"("Microscope Settings"=w320) -> ("Analogue Out out"=w322:waveform(dbl)[], "Digital Out out"=w323:digitalwaveform[])  [unwired: 2 in]
                }
                frame "Tweezers" {
                  n45 = Bundle By Name(cluster=w336, "Colour"=T13 [{"Laser"=enum."561", "Filter"=4}]) -> (w334:T2)
                  n46 = Bundle By Name(cluster=w334, "Colour"=T13 [{"Laser"=enum."488", "Filter"=4}], "ROI.Z"="Tweezers") -> (w333:T2)
                  n47 = call "XYZWaveforms.vi"("Microscope Settings"=w334) -> ("Analogue Out out"=w329:waveform(dbl)[], "Digital Out out"=w332:digitalwaveform[])  [unwired: 2 in]
                  n48 = call "XYZWaveforms.vi"("Microscope Settings"=w333) -> ("Analogue Out out"=w328:waveform(dbl)[], "Digital Out out"=w331:digitalwaveform[])  [unwired: 2 in]
                  n49 = for {
                    tunnel: w331 -> [w344] mode=indexing
                    tunnel: w332 -> [w345] mode=indexing
                    tunnel: [w343] -> w330 mode=indexing
                    n50 = call-poly <vilib>:"Append Digital Samples.vi"("digital waveform B"=w344, "digital waveform A"=w345) -> ("digital waveform out"=w343:digitalwaveform)  [unwired: 8 in, 1 out]
                  }
                  n51 = for {
                    tunnel: w328 -> [w341] mode=indexing
                    tunnel: w329 -> [w342] mode=indexing
                    tunnel: [w340] -> w327 mode=indexing
                    n52 = call-poly <vilib>:"Append Waveforms.vi"("waveform B"=w341, "waveform A"=w342) -> ("waveform out"=w340:waveform(dbl))  [unwired: 8 in, 1 out]
                  }
                }
              }
              n53 = Bundle By Name(cluster=w265, "Calibration Coordinates.Waveforms.Analogue Out"=w261, "Calibration Coordinates.Waveforms.Digital Out"=w262) -> (w264:T2)
              n54 = Bundle(Hardware."Update", "Microscope Settings"=w264) -> (w259:cluster{T12, "Microscope Settings":T2})  [unwired: 1 in]
              n55 = Enqueue Element(queue=w263, element=w259) -> ()  [unwired: 2 in, 3 out]
              n56 = Bundle("Analogue Out out"=w261, "Digital Out out"=w262) -> (w260:T18)  [unwired: 1 in]
              n57 = Index Array(array=w261) -> (element=w276:waveform(dbl))  [unwired: 1 in]
              n58 = call-poly <vilib>:"Waveform Duration.vi"("waveform in"=w276) -> ("duration"=w274:dbl)  [unwired: 8 in, 2 out]
              n59 = call "Graph.vi"("Cluster"=w260) -> ()
              n60 = To Time Stamp(1:w274) -> (0:w275:timestamp)
              n61 = Format Date/Time String(time format string (%c)="%H:%M:%S%4u", seconds (now)=w275) -> (date/time string=w271:string)  [unwired: 1 in]
              "Waveform Duration" <- w271
              n62 = property on="Waveform Duration" class="Str"("Value"=w271) -> ()  [unwired: 2 in, 2 out]
            }
            frame "runWaves" {
              n63 = Bundle(Hardware."Run Waves", "Microscope Settings"=w348) -> (w347:cluster{T12, "Microscope Settings":T2})  [unwired: 1 in]
              n64 = Enqueue Element(queue=w351, element=w347) -> ()  [unwired: 2 in, 3 out]
            }
            frame "runWavesCont" {
              n65 = Bundle(Hardware."RunCont", "Microscope Settings"=w357) -> (w356:cluster{T12, "Microscope Settings":T2})  [unwired: 1 in]
              n66 = Enqueue Element(queue=w360, element=w356) -> ()  [unwired: 2 in, 3 out]
            }
            frame "endWavesCont" {
              n67 = Bundle(Hardware."EndCont", "Microscope Settings"=w367) -> (w366:cluster{T12, "Microscope Settings":T2})  [unwired: 1 in]
              n68 = Enqueue Element(queue=w370, element=w366) -> ()  [unwired: 2 in, 3 out]
            }
            frame "stop" {
            }
          }
          n69 = local read "stop"() -> (w239:bool)
          n70 = Or(x=w240, y=w239) -> (x .or. y?=w238:bool)
          "Numeric 3" <- w233
        }
        n71 = call "IMAQ Create"("Image Name"="Images", "Image Type"=w119) -> ("New Image"=w129:T3, "error out"=w127:errorcluster)  [unwired: 3 in]
        n72 = while {
          tunnel: w139 -> [w698]
          shift-right: [w697] -> _
          shift-left: _ -> [w696]
          tunnel: w126 -> [w694]
          shift-right: [w693] -> _
          shift-left: w134 -> [w692]
          shift-right: [w691] -> w133
          shift-left: w132 -> [w690]
          stop <- w699 stop-if-true
          n73 = event shown="[16] \"Load Settings\": Value Change" {
            selector: _ -> [_ _ _ _ _ _ _ _ _ _ _ _ _ _ _ _ _]
            dyn-events: _ -> [_ _ _ _ _ _ _ _ _ _ _ _ _ _ _ _ _]
            timeout: 1 -> [_ _ _ _ _ _ _ _ _ _ _ _ _ _ _ _ _]
            tunnel: [w712 _ _ _ _ _ _ _ _ _ _ _ _ _ _ _ _] -> w699
            tunnel: w698 -> [w707 _ w731 w737 w748 _ w762 _ _ _ w798 _ _ _ _ _ _]
            tunnel: [w705 _ w725 w736 _ _ _ _ _ _ _ _ _ _ w852 _ w875] -> w697
            tunnel: w696 -> [w705 w719 w725 w736 w744 w753 w761 w775 w782 w788 w799 _ w819 w837 _ w856 w876]
            tunnel: w694 -> [w706 _ w730 _ w745 w754 _ w774 w778 w789 w797 _ w818 w836 _ _ _]
            tunnel: [w704 w714 w724 w734 w747 w757 w763 w773 w784 w791 w796 w807 w816 w834 w851 w857 w877] -> w693
            tunnel: w692 -> [w704 w716 w724 w734 w747 w757 w763 w773 w784 w791 w796 w807 w816 w834 w851 w857 w877]
            tunnel: [w700 w713 w720 w732 w739 w751 w759 w771 w780 w786 w792 w805 w815 w833 w850 w855 _] -> w691
            tunnel: w690 -> [w703 w713 w723 w733 w742 w752 w760 w772 w781 w785 w795 w804 w814 w832 w850 w853 _]
            event "stop": Value Change {
              w710 = ModeEnum."stop"  # Mode
              n74 = event-data() -> ()  [unwired: 1 in, 6 out]
              n75 = Bundle("Enum"=CameraControlTypeDef."Idle", "Value"=w705) -> (w708:cluster{"Enum":T11, "Value":T2})  [unwired: 1 in]
              n76 = Bundle("Mode"=w710, "Value"=w705) -> (w709:cluster{"Mode":T10, "Value":T2})  [unwired: 1 in]
              n77 = Enqueue Element(queue=w707, element=w708, error in (no error)=w703) -> (error out=w701:errorcluster)  [unwired: 1 in, 2 out]
              n78 = Enqueue Element(queue=w706, element=w709, error in (no error)=w703) -> (error out=w702:errorcluster)  [unwired: 1 in, 2 out]
              n79 = Merge Errors(w701, w702) -> (w700:errorcluster)
              n80 = local read "stop"() -> (w712:bool)
            }
            event Value Change {
              n81 = event-data() -> ()  [unwired: 1 in, 6 out]
              n82 = Flatten To XML(anything=w719) -> (xml string=w718:string)
              n83 = Build Array("Experiment 1" ("element"), w718) -> (w715:string[])
              n84 = Build Array (concatenate)(w716, w715) -> (w714:string[][])
              n85 = property on="Multicolumn Listbox" class="MCListbox (strict)"("ItemNames"=w714) -> ()  [unwired: 2 in, 2 out]
            }
            event Value Change {
              w728 = ModeEnum."generateWaves"  # Mode
              # "Live video for Calibration and 2D\nScan Modes.\n\nIdle Video for MultiD Scan modes\nUNTIL Begin Scan Button pressed?\n\nMultiD is waiting for trigger"
              n86 = event-data() -> ()  [unwired: 1 in, 6 out]
              n87 = Bundle("Enum"=CameraControlTypeDef."Trigger Source", "Value"=w725) -> (w726:cluster{"Enum":T11, "Value":T2})  [unwired: 1 in]
              n88 = Bundle("Mode"=w728, "Value"=w725) -> (w727:cluster{"Mode":T10, "Value":T2})  [unwired: 1 in]
              n89 = Enqueue Element(queue=w731, element=w726, error in (no error)=w723) -> (error out=w721:errorcluster)  [unwired: 1 in, 2 out]
              n90 = Enqueue Element(queue=w730, element=w727, error in (no error)=w723) -> (error out=w722:errorcluster)  [unwired: 1 in, 2 out]
              n91 = Merge Errors(w721, w722) -> (w720:errorcluster)
            }
            event Value Change {
              n92 = event-data() -> ()  [unwired: 1 in, 6 out]
              n93 = Bundle("Enum"=CameraControlTypeDef."Readout Mode", "Value"=w736) -> (w735:cluster{"Enum":T11, "Value":T2})  [unwired: 1 in]
              n94 = Enqueue Element(queue=w737, element=w735, error in (no error)=w733) -> (error out=w732:errorcluster)  [unwired: 1 in, 2 out]
            }
            event Value Change {
              w743 = ModeEnum."generateWaves"  # Mode
              n95 = event-data() -> ()  [unwired: 1 in, 6 out]
              n96 = Bundle("Enum"=CameraControlTypeDef."ROI", "Value"=w744) -> (w749:cluster{"Enum":T11, "Value":T2})  [unwired: 1 in]
              n97 = Bundle("Mode"=w743, "Value"=w744) -> (w746:cluster{"Mode":T10, "Value":T2})  [unwired: 1 in]
              n98 = Enqueue Element(queue=w748, element=w749, error in (no error)=w742) -> (error out=w740:errorcluster)  [unwired: 1 in, 2 out]
              n99 = Enqueue Element(queue=w745, element=w746, error in (no error)=w742) -> (error out=w741:errorcluster)  [unwired: 1 in, 2 out]
              n100 = Merge Errors(w740, w741) -> (w739:errorcluster)
            }
            event Value Change {
              w755 = ModeEnum."generateWaves"  # Mode
              n101 = event-data() -> ()  [unwired: 1 in, 6 out]
              n102 = Bundle("Mode"=w755, "Value"=w753) -> (w756:cluster{"Mode":T10, "Value":T2})  [unwired: 1 in]
              n103 = Enqueue Element(queue=w754, element=w756, error in (no error)=w752) -> (error out=w751:errorcluster)  [unwired: 1 in, 2 out]
            }
            event "Record": Value Change {
              n104 = event-data() -> ()  [unwired: 1 in, 6 out]
              n105 = case shown="True" "Record" {
                tunnel: w762 -> [_ w770]
                tunnel: w761 -> [_ w768]
                tunnel: w760 -> [w764 w766]
                tunnel: [w764 w765] -> w759
                frame False {
                }
                frame True {
                  n106 = Bundle("Enum"=CameraControlTypeDef."Ram Record", "Value"=w768) -> (w767:cluster{"Enum":T11, "Value":T2})  [unwired: 1 in]
                  n107 = Enqueue Element(queue=w770, element=w767, error in (no error)=w766) -> (error out=w765:errorcluster)  [unwired: 1 in, 2 out]
                }
              }
            }
            event Value Change {
              w777 = ModeEnum."generateWaves"  # Mode
              n108 = event-data() -> ()  [unwired: 1 in, 6 out]
              n109 = Bundle("Mode"=w777, "Value"=w775) -> (w776:cluster{"Mode":T10, "Value":T2})  [unwired: 1 in]
              n110 = Enqueue Element(queue=w774, element=w776, error in (no error)=w772) -> (error out=w771:errorcluster)  [unwired: 1 in, 2 out]
            }
            event Value Change {
              w783 = ModeEnum."generateWaves"  # Mode
              n111 = event-data() -> ()  [unwired: 1 in, 6 out]
              n112 = Bundle("Mode"=w783, "Value"=w782) -> (w779:cluster{"Mode":T10, "Value":T2})  [unwired: 1 in]
              n113 = Enqueue Element(queue=w778, element=w779, error in (no error)=w781) -> (error out=w780:errorcluster)  [unwired: 1 in, 2 out]
            }
            event Value Change {
              w790 = ModeEnum."generateWaves"  # Mode
              n114 = event-data() -> ()  [unwired: 1 in, 6 out]
              n115 = Bundle("Mode"=w790, "Value"=w788) -> (w787:cluster{"Mode":T10, "Value":T2})  [unwired: 1 in]
              n116 = Enqueue Element(queue=w789, element=w787, error in (no error)=w785) -> (error out=w786:errorcluster)  [unwired: 1 in, 2 out]
            }
            event Value Change {
              w802 = ModeEnum."generateWaves"  # Mode
              n117 = event-data() -> ()  [unwired: 1 in, 6 out]
              n118 = Bundle("Enum"=CameraControlTypeDef."Update", "Value"=w799) -> (w800:cluster{"Enum":T11, "Value":T2})  [unwired: 1 in]
              n119 = Bundle("Mode"=w802, "Value"=w799) -> (w801:cluster{"Mode":T10, "Value":T2})  [unwired: 1 in]
              n120 = Enqueue Element(queue=w798, element=w800, error in (no error)=w795) -> (error out=w794:errorcluster)  [unwired: 1 in, 2 out]
              n121 = Enqueue Element(queue=w797, element=w801, error in (no error)=w795) -> (error out=w793:errorcluster)  [unwired: 1 in, 2 out]
              n122 = Merge Errors(w794, w793) -> (w792:errorcluster)
            }
            event "Signals Debugger": Value Change {
              n123 = event-data() -> ()  [unwired: 1 in, 6 out]
              n124 = case shown="True" "Signals Debugger" {
                tunnel: [w808 w810] -> w805
                tunnel: w804 -> [w808 w809]
                frame False {
                }
                frame True {
                  n125 = vi-ref "Graph.vi"() -> (w811:refnum<vi>)
                  n126 = invoke class="VI" method="FP.Open"(reference=w811, error in=w809, "Activate"=TRUE ("Front Panel Window:Open"), "State"=T14."Standard") -> (error out=w810:errorcluster)  [unwired: 1 in, 4 out]
                }
              }
            }
            event "Scan": Value Change {
              n127 = event-data() -> ("NewVal"=w817:bool)  [unwired: 1 in, 5 out]
              n128 = case shown="True" w817 {
                tunnel: w819 -> [_ w825]
                tunnel: w818 -> [_ w824]
                tunnel: [w820 w823] -> w815
                tunnel: w814 -> [w820 w822]
                frame False {
                }
                frame True {
                  n129 = for {
                    N: "Scans" -> [_]
                    tunnel: w825 -> [w828]
                    tunnel: w824 -> [w831]
                    tunnel: [w827] -> w823
                    tunnel: w822 -> [w826]
                    w830 = ModeEnum."runWaves"  # Mode
                    n130 = Bundle("Mode"=w830, "Value"=w828) -> (w829:cluster{"Mode":T10, "Value":T2})  [unwired: 1 in]
                    n131 = Enqueue Element(queue=w831, element=w829, error in (no error)=w826) -> (error out=w827:errorcluster)  [unwired: 1 in, 2 out]
                  }
                }
              }
            }
            event "Scan Cont": Value Change {
              n132 = event-data() -> ("NewVal"=w835:bool)  [unwired: 1 in, 5 out]
              n133 = case shown="True" w835 {
                tunnel: w837 -> [w843 w849]
                tunnel: w836 -> [w842 w848]
                tunnel: [w841 w847] -> w833
                tunnel: w832 -> [w840 w846]
                frame True {
                  w839 = ModeEnum."runWavesCont"  # Mode
                  n134 = Bundle("Mode"=w839, "Value"=w843) -> (w838:cluster{"Mode":T10, "Value":T2})  [unwired: 1 in]
                  n135 = Enqueue Element(queue=w842, element=w838, error in (no error)=w840) -> (error out=w841:errorcluster)  [unwired: 1 in, 2 out]
                }
                frame False {
                  w845 = ModeEnum."endWavesCont"  # Mode
                  n136 = Bundle("Mode"=w845, "Value"=w849) -> (w844:cluster{"Mode":T10, "Value":T2})  [unwired: 1 in]
                  n137 = Enqueue Element(queue=w848, element=w844, error in (no error)=w846) -> (error out=w847:errorcluster)  [unwired: 1 in, 2 out]
                }
              }
            }
            event Timeout {
              n138 = event-data() -> ()  [unwired: 1 in, 3 out]
              n139 = property on="Microscope Settings" class="Clust (strict)"() -> ("Value"=w852:T2)  [unwired: 2 in, 2 out]
            }
            event "Save Settings": Value Change {
              n140 = event-data() -> ("NewVal"=w854:bool)  [unwired: 1 in, 5 out]
              n141 = case shown="True" w854 {
                tunnel: w856 -> [_ w873]
                tunnel: [w858 w861] -> w855
                tunnel: w853 -> [w858 _]
                frame False {
                }
                frame True {
                  n142 = Flatten To XML(anything=w873) -> (xml string=w866:string)
                  n143 = call "File Dialog"("start path"=path "C:/_DATA", "prompt"="Save your Settings", "button label"="Save", "default name"="SpimSettings", "pattern (all files)"=".xml") -> ("selected path"=w867:path, "error out"=w860:errorcluster)  [unwired: 7 in, 2 out]
                  n144 = Open/Create/Replace File(file path (use dialog)=w867, error in=w860, operation (0:open)=T15."replace or create with confirmation") -> (refnum out=w865:refnum<file>, error out=w862:errorcluster)  [unwired: 3 in, 1 out]
                  n145 = Write to Text File(file (use dialog)=w865, text=w866, error in=w862) -> (refnum out=w864:refnum<file>, error out=w863:errorcluster)  [unwired: 1 in, 1 out]
                  n146 = Close File(refnum=w864, error in=w863) -> (error out=w861:errorcluster)  [unwired: 1 out]
                }
              }
            }
            event "Load Settings": Value Change {
              n147 = event-data() -> ("NewVal"=w874:bool)  [unwired: 1 in, 5 out]
              n148 = case shown="True" w874 {
                tunnel: w876 -> [w878 w881]
                tunnel: [w878 w880] -> w875
                frame False {
                }
                frame True {
                  (unwired) "Load your Settings" ("prompt")
                  n149 = call "File Open"("start path"=path "C:/_DATA", "button label"="Load", "default name"="SpimSettings", "pattern (all files)"="*.xml") -> ("selected path"=w882:path, "cancelled"=w879:bool)  [unwired: 8 in, 2 out]
                  n150 = case shown="False" w879 {
                    tunnel: w882 -> [_ w892]
                    tunnel: w881 -> [w887 w890]
                    tunnel: [w887 w888] -> w880
                    frame True {
                    }
                    frame False {
                      n151 = Read from Text File(file (use dialog)=w892) -> (text=w891:string, error out=w889:errorcluster)  [unwired: 3 in, 2 out]
                      n152 = Unflatten From XML(xml string=w891, type=w890, error in (no error)=w889) -> (value=w888:T2)  [unwired: 1 out]
                      n153 = property on="Microscope Settings" class="Clust (strict)"("Val(Sgnl)"=w888) -> ()  [unwired: 2 in, 2 out]
                    }
                  }
                }
              }
            }
          }
        }
        n154 = while "Camera Consumer" {
          tunnel: w132 -> [w460]
          tunnel: [w464] -> w148
          tunnel: w139 -> [w471]
          tunnel: [w478] -> w147
          shift-right: [w477] -> _
          shift-left: CameraControlTypeDef."Preview" ("Enum") -> [w468]
          tunnel: [w474] -> w143
          tunnel: w142 -> [w473]
          tunnel: w140 -> [w467]
          shift-right: [w475] -> w151
          shift-left: w152 -> [w476]
          tunnel: w126 -> [w462]
          i -> [w458]
          stop <- w463 stop-if-true
          n155 = Dequeue Element(queue=w471, timeout in ms (-1)=1, error in (no error)=w460) -> (queue out=w470:refnum<queue>, element=w466:cluster{"Enum":T11, "Microscope Settings":T2}, timed out?=w459:bool, error out=w461:errorcluster)
          n156 = case shown="False" w459 {
            tunnel: [w480 CameraControlTypeDef."Preview" ("Enum")] -> w469
            tunnel: w468 -> [_ _]
            tunnel: w466 -> [w481 _]
            tunnel: [w479 _] -> w465
            frame False {
              n157 = Unbundle(w481) -> ("Enum"=w480:T11, "Microscope Settings"=w479:T2)
            }
            frame True {
            }
          }
          n158 = case shown="\"Preview\"" w469 {
            selector: w469 -> [w486 w491 w525 w542 w547 w558 w563 w568 w573 w578 w611 w629 _ w658 _]
            tunnel: w470 -> [w485 w492 w526 w543 w548 w559 w564 w569 w574 w579 _ w625 w640 w660 w679]
            tunnel: [w485 w492 w526 w543 w548 w559 w564 w569 w574 w579 _ w625 w640 w660 w679] -> w478
            tunnel: w461 -> [w487 w490 w524 w541 w546 w557 w562 w567 w572 w577 w606 w628 w631 w657 w670]
            tunnel: [w487 w490 w501 w541 w546 w557 w562 w567 w572 w577 w580 w628 w634 w657 w671] -> w464
            tunnel: [w486 w491 w525 w542 w547 w558 w563 w568 w573 w578 w611 w629 CameraControlTypeDef."Preview" ("Enum") w658 w661] -> w477
            tunnel: w476 -> [w484 w489 w508 w540 w544 w555 w561 w566 w571 w576 w608 w627 w630 w659 w673]
            tunnel: [w484 w489 w507 w540 w544 w554 w561 w566 w571 w576 w582 w627 w638 w659 w672] -> w475
            tunnel: [w483 w488 w503 w539 w545 w556 w560 w565 w570 w575 w610 w626 w636 w656 w674] -> w474
            tunnel: w473 -> [w483 w488 _ w539 w545 w556 w560 w565 w570 w575 w610 w626 w636 w656 _]
            tunnel: w467 -> [_ _ w517 _ _ _ _ _ _ _ _ _ w635 _ _]
            tunnel: w465 -> [_ _ w496 _ _ w553 _ _ _ _ w605 _ _ _ w663]
            tunnel: w462 -> [_ _ w497 _ _ _ _ _ _ _ _ _ _ _ _]
            frame "Idle" {
            }
            frame "IntervalLineInt" {
            }
            frame "Ram Record" {
              w521 = 0 items=["Snap", "Sequence"] ("Capture mode")
              w504 = 1 items=["Snap", "Sequence"] ("Capture mode")
              n159 = call "tm_stopcapture.vi"("error in (no error)"=w524, "Handle in"=w508) -> ("error out"=w499:errorcluster, "Handle out"=w500:u32)  [unwired: 8 in]
              n160 = call "tm_unpreparecapture.vi"("error in (no error)"=w499, "Handle in"=w500) -> ("error out"=w523:errorcluster, "Handle out"=w522:u32)  [unwired: 8 in]
              n161 = call "tm_preparecapture.vi"("error in (no error)"=w523, "Frames"="Frames", "Capture mode"=w521, "Handle in"=w522) -> ("error out"=w519:errorcluster, "Buffer Info"=w505:T5, "Handle out"=w520:u32)  [unwired: 4 in, 1 out]
              n162 = Bundle("Mode"=ModeEnum."runWaves", "Microscope Settings"=w496) -> (w493:cluster{"Mode":T10, "Microscope Settings":T2})  [unwired: 1 in]
              n163 = call "tm_startcapture_b.vi"("error in (no error)"=w519, "Handle in"=w520) -> ("error out"=w495:errorcluster, "Handle out"=w518:u32)  [unwired: 8 in]
              n164 = Enqueue Element(queue=w497, element=w493, error in (no error)=w495) -> (error out=w494:errorcluster)  [unwired: 1 in, 2 out]
              n165 = for {
                N: "Frames" -> [_]
                tunnel: w495 -> [w538]
                tunnel: w518 -> [w537]
                tunnel: w517 -> [w533]
                tunnel: [w531] -> w513
                tunnel: [w530] -> w512
                tunnel: w505 -> [w529]
                tunnel: w495 -> [_]
                tunnel: w497 -> [_]
                tunnel: w496 -> [_]
                tunnel: w494 -> [_]
                n166 = call "tm_waitnextframe.vi"("error in (no error)"=w538, "Handle in"=w537) -> ("error out"=w536:errorcluster, "Handle out"=w535:u32)  [unwired: 6 in, 2 out]
                n167 = call "tm_getframe_a.vi"("error in (no error)"=w536, "Buffer Info"=w529, "Handle in"=w535) -> ("error out"=w531:errorcluster, "Data 16"=w527:u16[][], "Handle out"=w530:u32)  [unwired: 4 in, 2 out]
                n168 = Bundle By Name(cluster=T8 {"State"=enum."Start Sequence", "Stack Number"=0, "Image"=[], "Stacks"=0} ("element"), "State"=Stack_Track."Save Image", "Image"=w527) -> (w532:T8)
                n169 = Enqueue Element(queue=w533, element=w532) -> ()  [unwired: 2 in, 3 out]
              }
              n170 = call "tm_stopcapture.vi"("error in (no error)"=w513, "Handle in"=w512) -> ("error out"=w514:errorcluster, "Handle out"=w511:u32)  [unwired: 8 in]
              n171 = call "tm_unpreparecapture.vi"("error in (no error)"=w514, "Handle in"=w511) -> ("error out"=w515:errorcluster, "Handle out"=w510:u32)  [unwired: 8 in]
              n172 = call "tm_preparecapture.vi"("error in (no error)"=w515, "Capture mode"=w504, "Handle in"=w510) -> ("error out"=w516:errorcluster, "Buffer Info"=w503:T5, "Handle out"=w509:u32)  [unwired: 5 in, 1 out]
              n173 = call "tm_startcapture_b.vi"("error in (no error)"=w516, "Handle in"=w509) -> ("error out"=w502:errorcluster, "Handle out"=w507:u32)  [unwired: 8 in]
              n174 = Merge Errors(w494, w502) -> (w501:errorcluster)
            }
            frame "HardDisk Record" {
            }
            frame "Disengage Update" {
            }
            frame "Update", Default {
              w550 = u32 2049184 items=["SENSOR MODE"=4212128, "CCD MODE"=4212384, "READOUT MODE"=4211872, "ACTIVE VIEW INDEX"=4343136, "BITS PER CHANNEL"=4342976, "IMAGE PIXEL TYPE"=4343296, "BINNING"=4215968, "EXPOSURE TIME"=2049184, "CONTRAST GAIN"=3163312, "CONTRAST OFFSET"=3163328, "LIGHT MODE"=2114720, "SENSITIVITY"=2114992, "PHOTON IMAGING MODE"=2115200, "HIGH DYNAMIC RANGE MODE"=3163360, "WHITE BALANCE"=3163568, "TEMPERATURE"=2115232, "TEMPERATURE TARGET"=2115264, "SENSOR COOLER FAN"=2115296, "LINEBUNDLE HEIGHT"=4212192, "MECHANICAL SHUTTER"=2115488, "BACK FOCUS POSITION"=8422304, "TRIGGER CONNECTOR"=1066432, "TRIGGER SOURCE"=1066144, "OUTPUT TRIGGER SOURCE"=1852576, "TRIGGER GLOBAL EXPOSURE"=2049680, "FIRST TRIGGER BEHAVIOR"=2049696, "CHANNEL SYNC"=1852352, "READOUT DIRECTION"=4211904, "PRE HSYNC COUNT"=1852704, "INTERNAL LINE SPEED"=4226000, "INTERNAL LINE INTERVAL"=4226016] ("Parameter")
              n175 = Unbundle By Name(w553) -> ("Exposure/ms"=w552:dbl)  [unwired: 1 out]
              n176 = Divide(x=w552, y=1000.0) -> (x/y=w549:dbl)
              n177 = call "tm_setparameter_a.vi"("Value in"=w549, "Parameter"=w550, "Handle in"=w555) -> ("Handle out"=w554:u32)  [unwired: 7 in, 1 out]
            }
            frame "ROI" {
            }
            frame "Binning" {
            }
            frame "Scan Mode" {
            }
            frame "Trigger Mode" {
            }
            frame "Readout Mode" {
              w586 = 1 items=["Snap", "Sequence"] ("Capture mode")
              w592 = u32 4194832  # Sensor Mode
              w595 = u32 2031888  # Exposure time
              n178 = Unbundle By Name(w605) -> ("Exposure/ms"=w604:dbl, "Slit.Slit Width /%"=w600:dbl, "Slit.Scanning Mode"=w590:dbl)
              n179 = call "tm_stopcapture.vi"("error in (no error)"=w606, "Handle in"=w608) -> ("error out"=w609:errorcluster, "Handle out"=w607:u32)  [unwired: 8 in]
              n180 = Divide(x=w604, y=1000.0) -> (x/y=w602:dbl)
              n181 = Multiply(x=w600, y=2048 ("input variable")) -> (x*y=w599:dbl)
              n182 = call "tm_unpreparecapture.vi"("error in (no error)"=w609, "Handle in"=w607) -> ("error out"=w587:errorcluster, "Handle out"=w591:u32)  [unwired: 8 in]
              n183 = call "tm_setpropertyvalue.vi"("error in (no error)"=w587, "Value in"=w590, "Property ID"=w592, "Handle in"=w591) -> ("error out"=w588:errorcluster, "Handle out"=w589:u32)  [unwired: 6 in]
              n184 = Divide(x=w599, y=100.0) -> (x/y=w597:dbl)
              n185 = case shown="1, Default" w590 {
                tunnel: [w614 w615] -> w596
                tunnel: w602 -> [w614 w623]
                tunnel: w597 -> [_ w622]
                tunnel: w589 -> [w613 w617]
                tunnel: [w613 w619] -> w594
                tunnel: [w612 w618] -> w593
                tunnel: w588 -> [w612 w616]
                frame 1, Default {
                }
                frame 12 {
                  w621 = u32 4208720  # Line Interval
                  n186 = formula code="slitExpos=frameInter*LW/(LinesToReadout\n+10+LW);\nlineInter = slitExpos / LW;"("frameInter"=w623, "LW"=w622, "LinesToReadout"=2048 ("input variable")) -> ("slitExpos"=w615:dbl, "lineInter"=w620:dbl)
                  n187 = call "tm_setpropertyvalue.vi"("error in (no error)"=w616, "Value in"=w620, "Property ID"=w621, "Handle in"=w617) -> ("error out"=w618:errorcluster, "Handle out"=w619:u32)  [unwired: 6 in]
                }
              }
              n188 = call "tm_setpropertyvalue.vi"("error in (no error)"=w593, "Value in"=w596, "Property ID"=w595, "Handle in"=w594) -> ("error out"=w581:errorcluster, "Handle out"=w583:u32)  [unwired: 6 in]
              n189 = call "tm_preparecapture.vi"("error in (no error)"=w581, "Capture mode"=w586, "Handle in"=w583) -> ("error out"=w585:errorcluster, "Handle out"=w584:u32)  [unwired: 5 in, 2 out]
              n190 = call "tm_startcapture_b.vi"("error in (no error)"=w585, "Handle in"=w584) -> ("error out"=w580:errorcluster, "Handle out"=w582:u32)  [unwired: 8 in]
            }
            frame "Readout Direction" {
            }
            frame "Preview" {
              n191 = call "tm_waitnextframe.vi"("error in (no error)"=w631, "Timeout"=500, "Handle in"=w630) -> ("error out"=w633:errorcluster, "Handle out"=w639:u32)  [unwired: 5 in, 2 out]
              n192 = case shown="No Error" w633 {
                selector: w633 -> [w641 w655]
                tunnel: w639 -> [w653 w654]
                tunnel: [w652 w654] -> w638
                tunnel: w636 -> [w651 _]
                tunnel: w635 -> [w650 _]
                tunnel: w631 -> [w645 _]
                tunnel: [w642 w655] -> w634
                frame No Error {
                  w647 = 0 ("Timeout")
                  n193 = call "tm_getframe_a.vi"("error in (no error)"=w641, "Buffer Info"=w651, "Handle in"=w653) -> ("error out"=w643:errorcluster, "Data 16"=w648:u16[][], "Handle out"=w652:u32)  [unwired: 4 in, 2 out]
                  n194 = Bundle("State"=Stack_Track."Display", "Timeout"=w647, "Data 16"=w648, "Timeout"=w647) -> (w646:T19)  [unwired: 1 in]
                  n195 = Enqueue Element(queue=w650, element=w646, error in (no error)=w645) -> (error out=w644:errorcluster)  [unwired: 1 in, 2 out]
                  n196 = Merge Errors(w643, w644) -> (w642:errorcluster)
                }
                frame Error {
                }
              }
            }
            frame "ROIWindow" {
            }
            frame "Trigger Source" {
              (unwired) u32 1066144 items=["SENSOR MODE"=4212128, "CCD MODE"=4212384, "READOUT MODE"=4211872, "ACTIVE VIEW INDEX"=4343136, "BITS PER CHANNEL"=4342976, "IMAGE PIXEL TYPE"=4343296, "BINNING"=4215968, "EXPOSURE TIME"=2049184, "CONTRAST GAIN"=3163312, "CONTRAST OFFSET"=3163328, "LIGHT MODE"=2114720, "SENSITIVITY"=2114992, "PHOTON IMAGING MODE"=2115200, "HIGH DYNAMIC RANGE MODE"=3163360, "WHITE BALANCE"=3163568, "TEMPERATURE"=2115232, "TEMPERATURE TARGET"=2115264, "SENSOR COOLER FAN"=2115296, "LINEBUNDLE HEIGHT"=4212192, "MECHANICAL SHUTTER"=2115488, "BACK FOCUS POSITION"=8422304, "TRIGGER CONNECTOR"=1066432, "TRIGGER SOURCE"=1066144, "OUTPUT TRIGGER SOURCE"=1852576, "TRIGGER GLOBAL EXPOSURE"=2049680, "FIRST TRIGGER BEHAVIOR"=2049696, "CHANNEL SYNC"=1852352, "READOUT DIRECTION"=4211904, "PRE HSYNC COUNT"=1852704, "INTERNAL LINE SPEED"=4226000, "INTERNAL LINE INTERVAL"=4226016] ("Parameter")
              w669 = 1 items=["Snap", "Sequence"] ("Capture mode")
              n197 = Unbundle By Name(w663) -> ("Mode"=w662:T17)
              n198 = call "tm_stopcapture.vi"("error in (no error)"=w670, "Handle in"=w673) -> ("error out"=w677:errorcluster, "Handle out"=w678:u32)  [unwired: 8 in]
              n199 = call "tm_unpreparecapture.vi"("error in (no error)"=w677, "Handle in"=w678) -> ("error out"=w665:errorcluster, "Handle out"=w668:u32)  [unwired: 8 in]
              n200 = case shown="\"XY\", Default" w662 {
                tunnel: [T7 {"Mode"=2, "Polarity"=2, "Times"=2, "Delay"=0.0} ("Parameters") T7 {"Mode"=2, "Polarity"=2, "Times"=2, "Delay"=0.0} ("Parameters") T7 {"Mode"=2, "Polarity"=2, "Times"=2, "Delay"=0.0} ("Parameters") T7 {"Mode"=1, "Polarity"=2, "Times"=2, "Delay"=0.0} ("Parameters") T7 {"Mode"=1, "Polarity"=2, "Times"=2, "Delay"=0.0} ("Parameters")] -> w666
                tunnel: [CameraControlTypeDef."Preview" ("Enum") CameraControlTypeDef."Idle" ("Enum") CameraControlTypeDef."Idle" ("Enum") CameraControlTypeDef."Idle" ("Enum") CameraControlTypeDef."Preview" ("Enum")] -> w661
                frame "XY", Default {
                }
                frame "XYZT" {
                }
                frame "XYZ" {
                }
                frame "XYZC" {
                }
                frame "X" {
                }
              }
              n201 = call "tm_setinputtrigger.vi"("error in (no error)"=w665, "Parameters"=w666, "Handle in"=w668) -> ("error out"=w664:errorcluster, "Handle out"=w667:u32)  [unwired: 7 in]
              n202 = call "tm_preparecapture.vi"("error in (no error)"=w664, "Capture mode"=w669, "Handle in"=w667) -> ("error out"=w676:errorcluster, "Buffer Info"=w674:T5, "Handle out"=w675:u32)  [unwired: 5 in, 1 out]
              n203 = call "tm_startcapture_b.vi"("error in (no error)"=w676, "Handle in"=w675) -> ("error out"=w671:errorcluster, "Handle out"=w672:u32)  [unwired: 8 in]
            }
          }
          n204 = local read "stop"() -> (w463:bool)
          "Frames" <- w458
        }
        n205 = while "Tiff Consumer" {
          tunnel: [w396] -> w146
          tunnel: w140 -> [w397]
          shift-right: [w390] -> _
          shift-left: w129 -> [w387]
          shift-right: [w385] -> _
          shift-left: u32[] [] -> [w386]
          shift-right: [w388] -> w149
          shift-left: w127 -> [w384]
          shift-right: [w381] -> _
          shift-left: T8 {"State"=enum."Idle", "Stack Number"=0, "Image"=[], "Stacks"=0} ("input cluster") -> [w380]
          i -> [w383]
          stop <- w399 stop-if-true
          # "Delay, maybe?\nCheck"
          n206 = Unbundle By Name(w380) -> ("State"=w392:T9, "Stack Number"=→"Stack Number":i32, "Image"=w393:u16[][])
          n207 = Dequeue Element(queue=w397, timeout in ms (-1)=1, error in (no error)=w384) -> (queue out=w395:refnum<queue>, element=w381:T8, error out=w394:errorcluster)  [unwired: 1 out]
          n208 = case shown="\"Save Image\"" w392 {
            tunnel: [w412 w428 w431 w436 w440 w444 w448 w457] -> w396
            tunnel: w395 -> [w412 w428 w431 w436 w440 w444 w448 w457]
            tunnel: w393 -> [w402 _ _ _ _ _ _ w456]
            tunnel: w387 -> [w400 w426 w430 w434 w438 w442 w446 w454]
            tunnel: w394 -> [w411 w427 w432 w435 w439 w443 w447 w455]
            tunnel: [w410 w427 w432 w435 w439 w443 w447 w450] -> w389
            tunnel: [w401 w426 w430 w434 w438 w442 w446 w451] -> w390
            tunnel: w386 -> [w409 w425 w429 w433 w437 w441 w445 w449]
            tunnel: [w404 w425 w429 w433 w437 w441 w445 w449] -> w385
            frame "Display" {
              w405 = 10 ("y")
              n209 = Add Array Elements(numeric array=w402) -> ()  [unwired: 1 out]
              n210 = call "IMAQ ArrayToImage"("Image Pixels (U16)"=w402, "error in (no error)"=w411, "Image"=w400) -> ("error out"=w410:errorcluster, "Image Out"=w401:T3)  [unwired: 7 in]
              n211 = Tick Count (ms)() -> (millisecond timer value=w403:u32)
              n212 = Build Array (concatenate)(w409, w403) -> (w406:u32[])
              n213 = Array Size(array=w406) -> (size(s)=w408:i32)
              n214 = Greater?(x=w408, y=w405) -> (0:w407:bool)
              n215 = case shown="True" w407 {
                tunnel: w406 -> [w413 w416]
                tunnel: w405 -> [_ w423]
                tunnel: [w413 w414] -> w404
                frame False {
                }
                frame True {
                  n216 = Array Subset(array=w416, index=1, length=w423) -> (w414:u32[])
                  n217 = Index Array(array=w414, index=0) -> (element=w420:u32)
                  n218 = Index Array(array=w414, index=9) -> (element=w421:u32)
                  n219 = Subtract(x=w421, y=w420) -> (x-y=w419:u32)
                  n220 = Divide(x=10000.0, y=w419) -> (x/y=→"FPS":dbl)
                }
              }
            }
            frame "Idle", Default {
            }
            frame "Start Sequence" {
            }
            frame "Read Disk" {
            }
            frame "STOP" {
            }
            frame "Collecting" {
            }
            frame "End" {
            }
            frame "Save Image" {
              n221 = call "4Digit File Incrementer.vi"("path"="Save to:") -> ("appended path"=w452:path)  [unwired: 10 in]
              n222 = call "IMAQ ArrayToImage"("Image Pixels (U16)"=w456, "error in (no error)"=w455, "Image"=w454) -> ("error out"=w450:errorcluster, "Image Out"=w451:T3)  [unwired: 7 in]
              n223 = local write "Save to:"(w452) -> ()
              n224 = call-poly "IMAQ Write File 2"("error in (no error)"=w450, "File Path"=w452, "Image"=w451) -> ()  [unwired: 7 in, 2 out]
            }
          }
          "Image" <- w390
          n225 = call "IMAQ Histograph"("error in (no error)"=w389, "Image"=w390) -> ("error out"=w388:errorcluster, "Histogram Graph"=→"Histogram":T4)  [unwired: 6 in, 2 out]
          n226 = local read "stop"() -> (w399:bool)
          "Numeric" <- w383
        }
        n227 = while {
          tunnel: [w176] -> w121
          tunnel: w120 -> [w175]
          shift-right: [w172] -> _
          shift-left: w123 -> [w170]
          shift-right: [w171] -> _
          shift-left: w122 -> [w169]
          shift-right: [w163] -> _
          shift-left: w124 -> [w165]
          shift-right: [w164] -> _
          shift-left: w125 -> [w166]
          shift-right: [w158] -> _
          shift-left: _ -> [w160]
          shift-right: [w155] -> _
          shift-left: _ -> [w153]
          i -> [w162]
          stop <- w168 stop-if-true
          n228 = Dequeue Element(queue=w175, timeout in ms (-1)=1) -> (queue out=w174:refnum<queue>, element=w173:cluster{T12, "Microscope Settings":T2}, timed out?=w159:bool)  [unwired: 1 in, 1 out]
          n229 = case shown="\"RunCont\"" w160 {
            tunnel: [w188 w196 w198 w210 w215 w228] -> w176
            tunnel: w174 -> [w188 w196 w198 w210 w215 w228]
            tunnel: w153 -> [_ w192 w202 _ w219 _]
            tunnel: [w187 w191 w203 w212 w220 w230] -> w172
            tunnel: [w186 w190 w204 w213 w221 w229] -> w171
            tunnel: w170 -> [w187 _ w203 w212 w220 w230]
            tunnel: w169 -> [w186 _ w204 w213 w221 w229]
            tunnel: [FALSE FALSE FALSE FALSE FALSE FALSE] -> w167
            tunnel: w166 -> [w185 w195 w206 w209 w223 w226]
            tunnel: w165 -> [w184 w194 w205 w208 w222 w225]
            tunnel: [w185 w195 w201 w209 w218 w226] -> w164
            tunnel: [w184 w194 w200 w208 w217 w225] -> w163
            tunnel: [Hardware."Idle" Hardware."Idle" Hardware."Idle" Hardware."Idle" Hardware."RunCont" Hardware."Idle"] -> w157
            frame "Idle", Default {
            }
            frame "Update" {
              n230 = Unbundle By Name(w192) -> ("Calibration Coordinates.Waveforms.Analogue Out"=w191:waveform(dbl)[], "Calibration Coordinates.Waveforms.Digital Out"=w190:digitalwaveform[])
              n231 = Bundle("Analogue Out"=w191, "Digital Out"=w190) -> ()  [unwired: 1 in, 1 out]
            }
            frame "Run Waves" {
              n232 = call "RunWaves.vi"("Analogue Out"=w203, "Digital Out"=w204, "Microscope Settings"=w202, "Mirror Z in"=w205, "Refnum in"=w206) -> ("task out"=w200:refnum<k21>, "Refnum out"=w201:refnum<k21>)  [unwired: 5 in]
            }
            frame "EndCont" {
            }
            frame "RunCont" {
              n233 = call "RunWaves.vi"("Analogue Out"=w220, "Digital Out"=w221, "Microscope Settings"=w219, "Mirror Z in"=w222, "Refnum in"=w223) -> ("task out"=w217:refnum<k21>, "Refnum out"=w218:refnum<k21>)  [unwired: 5 in]
            }
            frame "Stop" {
            }
          }
          n234 = Unbundle(w173) -> (w154:T12, "Microscope Settings"=w156:T2)
          n235 = case shown="True" w159 {
            tunnel: [w178 w181] -> w158
            tunnel: w157 -> [_ w181]
            tunnel: [w179 w180] -> w155
            tunnel: w156 -> [w179 _]
            tunnel: w154 -> [w178 _]
            tunnel: w153 -> [_ w180]
            frame False {
            }
            frame True {
            }
          }
          n236 = local read "stop"() -> (w177:bool)
          n237 = Or(x=w167, y=w177) -> (x .or. y?=w168:bool)
          "Numeric 2" <- w162
        }
        n238 = Merge Errors(w133, w148, w149) -> (w150:errorcluster)
      }
      frame "deinit" {
        n239 = call <vilib>:"DAQmx Stop Task.vi"("task/channels in"=w904) -> ("task out"=w905:refnum<k21>)  [unwired: 13 in, 1 out]
        n240 = call <vilib>:"DAQmx Stop Task.vi"("task/channels in"=w906) -> ("task out"=w907:refnum<k21>)  [unwired: 13 in, 1 out]
        n241 = call <vilib>:"DAQmx Clear Task.vi"("task in"=w905) -> ("error out"=w901:errorcluster)  [unwired: 14 in]
        n242 = call "tm_stopcapture.vi"("error in (no error)"=w915, "Handle in"=w911) -> ("error out"=w918:errorcluster, "Handle out"=w917:u32)  [unwired: 8 in]
        n243 = call <vilib>:"DAQmx Clear Task.vi"("task in"=w907) -> ("error out"=w902:errorcluster)  [unwired: 14 in]
        n244 = call "tm_unpreparecapture.vi"("error in (no error)"=w918, "Handle in"=w917) -> ("error out"=w919:errorcluster, "Handle out"=w916:u32)  [unwired: 8 in]
        n245 = call "tm_closecamera.vi"("error in (no error)"=w919, "Handle in"=w916) -> ("error out"=w920:errorcluster)  [unwired: 9 in]
        n246 = Flush Queue(queue=w894) -> (queue out=w900:refnum<queue>)  [unwired: 1 in, 2 out]
        n247 = call "tm_deinitialize.vi"("error in (no error)"=w920) -> ("error out"=w897:errorcluster)  [unwired: 10 in]
        n248 = Release Queue(queue=w895, error in (no error)=w897) -> (error out=w913:errorcluster)  [unwired: 1 in, 2 out]
        n249 = Release Queue(queue=w900) -> (error out=w903:errorcluster)  [unwired: 2 in, 2 out]
        n250 = Flush Queue(queue=w899, error in (no error)=w897) -> (queue out=w898:refnum<queue>, error out=w896:errorcluster)  [unwired: 1 out]
        n251 = Release Queue(queue=w898, error in (no error)=w896) -> (error out=w912:errorcluster)  [unwired: 1 in, 2 out]
        n252 = Merge Errors(w913, w912, w903, w902, w901) -> (w914:errorcluster)
      }
    }
    n253 = Or(x="stop", y=w21) -> (x .or. y?=w22:bool)
  }
  "error IO" <- w6
